vi "ME_acquire_16_DeltaForce_Daq.vi"() -> ()   [LabVIEW 2015]
doc: "Use this template to build a producer/consumer design pattern. Use this template when you need to execute a process, such as data analysis, when a data source, such as a triggered acquisition, produces data at an uneven rate and you need to execute the process when the data becomes available."
uses:
  Mode.ctl
  oxford_driver/Oxford Drivers/BUSGEN.LLB/OxfordAddress.ctl
  <vilib>/Analysis/baseanly.llb/Mean (DBL).vi
  <vilib>/DAQmx/read.llb/DAQmx Read (Analog 1D DBL 1Chan NSamp).vi
  <vilib>/DAQmx/create/channels.llb/DAQmx Create Channel (AI-Voltage-Basic).vi
  <vilib>/DAQmx/configure/timing.llb/DAQmx Timing (Sample Clock).vi
  <vilib>/Utility/file.llb/Write Delimited Spreadsheet (DBL).vi
  <vilib>/DAQmx/miscellaneous.llb/DAQmx Fill In Error Info.vi
  <vilib>/express/express arith-compare/Formula/XNode/ExpressFormulaBlockNode.xnode
  <vilib>/Analysis/NI_AALBase.lvlib
panel:
  out "T array":dbl[](array[numeric])
  out "Averaged I(T)":dbl[][](array[numeric])
  in  "Averaged P(T)":dbl[][](array[numeric])
  out "remaining elements 2":T1(array[cluster])
  out "Actual mean":dbl format="%0.6f"
  in  "Averaged dt":dbl[][](array[numeric])
  in  "Averaged P(B)":dbl[][](array[numeric])
  out "LockInR":dbl
  out "deltaUaux":dbl
  out "Actual Voltage (V)":dbl caption="Actual AuxV" step=0.1
  in  "Stop":bool
  out "SaveSweep":bool=TRUE
  out "Measurement File_dn":path
  out "Measurement File_up":path
  out "Measurement File_average":path
  out "Actual Polarization":dbl
  in  "Reset IB?":bool
  in  "First?":bool
  in  "Save Period":dbl=1.0
  out "Averaged I(B)":dbl[][](array[numeric])
  out "P(uC/mm^2)":dbl[](array[numeric])
  in  "Sweep":bool
  out "Offset array":dbl[](array[numeric])
  in  "stop 2":bool
  in  "dB":dbl=0.005
  out "appended array":dbl[][](array[numeric])
  out "Actual B Field (T)":dbl
  out "Actual Temperature (K)":dbl
  out "Actual Current (pA)":dbl
  in  "Tab Control":T2(tab)
  in  "dt (K)":dbl=0.1
  in  "Max temperature (K)":dbl=20.0
  in  "Min Temperature (K)":dbl=4.5
  out "P(T)":cluster{"yi":dbl[], dbl[]}(graph)
  out "I(T)":cluster{dbl[], dbl[]}(graph)
  in  "Set temperature (K)":dbl=4.5
  in  "Temp Ramping Rate (K/min)":dbl=10.0
  in  "Heater Range":enum16{"Off", "Low", "Medium", "High"}(ring)
  in  "Heater On/Off":bool
  out "Setpoint Temperature (K)":dbl
  out "I(T) /Averaged/":cluster{"B array":dbl[], dbl[]}[](graph)
  out "P(T) /Averaged/":cluster{"B array":dbl[], dbl[]}[](graph)
  out "Up/Down 2":bool
  out "I(B) 3":cluster{dbl[], dbl[]}[](graph)
  out "I(B) /Averaged/":cluster{"B array":dbl[], dbl[]}[](graph)
  out "P(B) /Averaged/":cluster{"B array":dbl[], dbl[]}[](graph)
  out "P(B)":cluster{"yi":dbl[], dbl[]}(graph)
  in  "Set Field (T)":dbl
  in  "Go to Set":bool
  in  "Sweep Rate (T/min)":dbl=2.0 format="%.6f"
  in  "Field To Zero":bool
  out "Target Field":dbl
  in  "Min Field (T)":dbl
  in  "Max Field (T)":dbl=0.15
  in  "Threshold B (T)":dbl
  out "Up/Down":bool
  in  "Magnetic Field array (T)":dbl[](array[numeric])=[0.025, 0.05, 0.075, 0.1, 0.125, 0.15, 0.175, 0.2, 0.225, 0.25, 0.275, 0.3]
  in  "T Sweep Rate Array":dbl[](array[numeric])=[10.0, 20.0]
  in  "Max count array":i32[](array[numeric])=[2, 1, 0, 0, 0, 9, 10, 11, 12]
  in  "secs to wait":dbl=180.0
  out "Wait (s)":dbl
  in  "Directory":string
  out "Finished":bool=TRUE
  out "Step Rate":bool
  out "New":bool=TRUE
  in  "Temperature Array":dbl[](array[numeric])=[4.5, 5.0, 6.0, 7.0, 8.0, 9.0, 10.0, 11.0, 12.0]
  in  "Sweep Rate Array":dbl[](array[numeric])=[2.0, 1.0, 0.5, 0.1, 0.05, 9.0, 10.0, 11.0, 12.0]
  in  "Record ALL":bool
  in  "Max Countl":i32
  out "i":i32
  out "j":i32
  out "Step Temp":bool
  in  "FileName":string
  in  "Measure Noise":bool
  in  "Cycles":i32
  in  "maximum value":dbl=10.0 format="%0.2f"
  in  "minimum value":dbl=-10.0 format="%0.2f"
  in  "physical channels":tag="Dev1/ai1"
  out "PSD (pA/Hz^1/2) Peaks Removed":cluster{"f0":dbl, "df":dbl, "magnitude":dbl[]}(graph)
  out "PSD (pA/Hz^1/2)":cluster{"f0":dbl, "df":dbl, "magnitude":dbl[]}(graph)
  out "Current (pA) Filtered":waveform(dbl)(graph)
  out "Current (pA)":dbl[](graph)
  in  "Samples per channel":i32=1000
  in  "Rate":dbl=1000.0 format="%0.2f"
  in  "Cut-Off Frequency":dbl=100.0 caption="Lower Cut-Off"
  in  "Filter On":bool
  in  "Keithley (IV conv) averaging":i32=10
  in  "Lock_in_Amplifier":refnum<visa-resource-name>="GPIB0::5::INSTR"
  out "Dc offset":dbl
  in  "Calibrate":bool
  in  "IV converter":refnum<visa-resource-name>="GPIB0::20::INSTR"
  in  "Magnetic Field":refnum<visa-resource-name>="GPIB0::21::INSTR"
  out "Time Lag":dbl=0.0500025749206543
  in  "Lake Shore":refnum<visa-resource-name>="GPIB0::11::INSTR"
  in  "Temp Refresh (s)":dbl=0.1
  in  "Sampling rate (Hz)":dbl=10.0
  in  "Gain (V/A)":dbl=1000000000.0
  in  "Sample area (mm^2)":dbl=1.0
  out "B_V":cluster{dbl[], "Best Linear Fit":dbl[]}[](graph)=[{[-0.00769241141, -0.00768011662, -0.0029394633, 0.00271952438, 0.00937200583, 0.0154641889, 0.0217080684, 0.0281692221, 0.0344763397, 0.0407091529, 0.0473661569, 0.0541476438, 0.0611164384, 0.0676637725, 0.073937413, 0.0801511723, 0.0863882257, 0.0933787866, 0.0997676928, 0.106163316, 0.113953626, 0.118979018, 0.126030157, 0.132855724, 0.13883398, 0.14631074, 0.153030676, 0.159156864, 0.165801088, 0.17248087, 0.178555009, 0.185285367, 0.192834407, 0.198751051, 0.205413053, 0.212847389, 0.219477697, 0.225574642, 0.232225854, 0.239015189, 0.245675966, 0.252411162, 0.258453848, 0.265211852, 0.271251534, 0.277801221, 0.284008329, 0.291402813, 0.297970768, 0.304082546, 0.310761405, 0.317366634, 0.323522001, 0.330123184, 0.336841279, 0.343557963, 0.349608435, 0.356238003, 0.363590921, 0.370338319, 0.376962983], "Best Linear Fit"=[0.0, 0.0015, 0.0035, 0.0056, 0.0076, 0.0096, 0.0116, 0.0136, 0.0156, 0.0177, 0.0197, 0.0219, 0.0239, 0.0259, 0.0279, 0.0299, 0.032, 0.034, 0.036, 0.038, 0.04, 0.042, 0.0441, 0.046, 0.048, 0.05, 0.052, 0.054, 0.056, 0.058, 0.06, 0.0621, 0.0643, 0.0663, 0.0684, 0.0704, 0.0725, 0.0745, 0.0765, 0.0787, 0.0807, 0.0827, 0.0847, 0.0868, 0.0888, 0.0908, 0.0928, 0.0948, 0.0968, 0.0988, 0.1008, 0.1028, 0.1048, 0.1069, 0.1091, 0.1111, 0.1131, 0.1152, 0.1173, 0.1193, 0.1213]}, {[-0.00769241141, -0.00768011662, -0.0029394633, 0.00271952438, 0.00937200583, 0.0154641889, 0.0217080684, 0.0281692221, 0.0344763397, 0.0407091529, 0.0473661569, 0.0541476438, 0.0611164384, 0.0676637725, 0.073937413, 0.0801511723, 0.0863882257, 0.0933787866, 0.0997676928, 0.106163316, 0.113953626, 0.118979018, 0.126030157, 0.132855724, 0.13883398, 0.14631074, 0.153030676, 0.159156864, 0.165801088, 0.17248087, 0.178555009, 0.185285367, 0.192834407, 0.198751051, 0.205413053, 0.212847389, 0.219477697, 0.225574642, 0.232225854, 0.239015189, 0.245675966, 0.252411162, 0.258453848, 0.265211852, 0.271251534, 0.277801221, 0.284008329, 0.291402813, 0.297970768, 0.304082546, 0.310761405, 0.317366634, 0.323522001, 0.330123184, 0.336841279, 0.343557963, 0.349608435, 0.356238003, 0.363590921, 0.370338319, 0.376962983], "Best Linear Fit"=[0.002353460844818253, 0.002357267374965663, 0.003824997997530172, 0.005577049655813272, 0.007636692089275871, 0.009522863265806463, 0.01145600043639222, 0.013456406815525209, 0.015409122826751182, 0.01733883381400479, 0.019399876452181594, 0.021499459635718428, 0.023657034245452215, 0.025684122519169482, 0.027626473848249778, 0.02955028565017564, 0.03148130942513291, 0.03364562299316916, 0.03562366117513693, 0.037603778974812686, 0.040015698972850115, 0.04157158615356273, 0.04375465501257369, 0.04586788562152819, 0.0477187843918964, 0.050033627699098075, 0.05211415440778254, 0.05401085368533849, 0.056067939569859164, 0.05813603439385595, 0.06001661903361471, 0.06210037244704129, 0.06443759401357516, 0.0662694173922171, 0.06833200743687069, 0.07063371605572277, 0.07268649347515121, 0.0745741389696738, 0.07663338837489471, 0.07873540137051047, 0.08079761214887074, 0.08288286343195213, 0.08475371006132383, 0.08684602281837933, 0.08871593939391825, 0.09074375613756333, 0.09266550866283872, 0.09495487889775463, 0.09698835150804998, 0.09888058937557581, 0.10094839843403076, 0.10299341126621803, 0.10489914451207855, 0.10694290468187984, 0.10902286140750632, 0.11110238128028392, 0.11297563849525552, 0.11502818680688229, 0.1173046879946565, 0.11939371707962458, 0.12144474708765744]}]
  out "V_I":cluster{dbl[], "Best Linear Fit":dbl[]}[](graph)=[{[0.0, 0.012, 0.026, 0.04, 0.054, 0.068, 0.081, 0.096, 0.11, 0.124, 0.138, 0.153, 0.167, 0.18, 0.195, 0.208, 0.223, 0.236, 0.251, 0.265, 0.279, 0.292, 0.306, 0.32, 0.334, 0.348, 0.362, 0.375, 0.389, 0.403, 0.417, 0.432, 0.446, 0.46, 0.475, 0.489, 0.504, 0.517, 0.531, 0.546, 0.56, 0.574, 0.588, 0.602, 0.616, 0.63, 0.644, 0.658, 0.672, 0.685, 0.699, 0.713, 0.727, 0.742, 0.755, 0.77, 0.784, 0.799, 0.814, 0.827, 0.841], "Best Linear Fit"=[-0.00769241141, -0.00768011662, -0.0029394633, 0.00271952438, 0.00937200583, 0.0154641889, 0.0217080684, 0.0281692221, 0.0344763397, 0.0407091529, 0.0473661569, 0.0541476438, 0.0611164384, 0.0676637725, 0.073937413, 0.0801511723, 0.0863882257, 0.0933787866, 0.0997676928, 0.106163316, 0.113953626, 0.118979018, 0.126030157, 0.132855724, 0.13883398, 0.14631074, 0.153030676, 0.159156864, 0.165801088, 0.17248087, 0.178555009, 0.185285367, 0.192834407, 0.198751051, 0.205413053, 0.212847389, 0.219477697, 0.225574642, 0.232225854, 0.239015189, 0.245675966, 0.252411162, 0.258453848, 0.265211852, 0.271251534, 0.277801221, 0.284008329, 0.291402813, 0.297970768, 0.304082546, 0.310761405, 0.317366634, 0.323522001, 0.330123184, 0.336841279, 0.343557963, 0.349608435, 0.356238003, 0.363590921, 0.370338319, 0.376962983]}, {[0.0, 0.012, 0.026, 0.04, 0.054, 0.068, 0.081, 0.096, 0.11, 0.124, 0.138, 0.153, 0.167, 0.18, 0.195, 0.208, 0.223, 0.236, 0.251, 0.265, 0.279, 0.292, 0.306, 0.32, 0.334, 0.348, 0.362, 0.375, 0.389, 0.403, 0.417, 0.432, 0.446, 0.46, 0.475, 0.489, 0.504, 0.517, 0.531, 0.546, 0.56, 0.574, 0.588, 0.602, 0.616, 0.63, 0.644, 0.658, 0.672, 0.685, 0.699, 0.713, 0.727, 0.742, 0.755, 0.77, 0.784, 0.799, 0.814, 0.827, 0.841], "Best Linear Fit"=[-0.015941127780698654, -0.010342478990544012, -0.0038107220686969304, 0.0027210348531501527, 0.009252791774997235, 0.01578454869684432, 0.02184975155284518, 0.028848062540538483, 0.03537981946238557, 0.041911576384232645, 0.048443333306079736, 0.05544164429377303, 0.061973401215620116, 0.06803860407162098, 0.07503691505931429, 0.08110211791531513, 0.08810042890300844, 0.0941656317590093, 0.10116394274670261, 0.1076956996685497, 0.11422745659039678, 0.12029265944639762, 0.1268244163682447, 0.1333561732900918, 0.13988793021193888, 0.14641968713378595, 0.15295144405563305, 0.15901664691163392, 0.165548403833481, 0.1720801607553281, 0.17861191767717516, 0.18561022866486845, 0.19214198558671555, 0.19867374250856262, 0.20567205349625592, 0.212203810418103, 0.2192021214057963, 0.22526732426179719, 0.23179908118364426, 0.23879739217133758, 0.24532914909318465, 0.2518609060150317, 0.2583926629368788, 0.2649244198587259, 0.271456176780573, 0.27798793370242003, 0.28451969062426713, 0.29105144754611423, 0.2975832044679613, 0.3036484073239622, 0.31018016424580924, 0.3167119211676563, 0.3232436780895034, 0.3302419890771967, 0.3363071919331976, 0.3433055029208909, 0.34983725984273795, 0.35683557083043127, 0.36383388181812454, 0.3698990846741254, 0.3764308415959725]}]
  out "B0 (T)":dbl=0.0026443907573365636
  out "B/V (T/V)":dbl=0.3027997253900218
  out "I0 (A)":dbl=-0.008736391445912099
  out "V/I (Ohm)":dbl=0.4773805959957447
  in  "Offset?":bool
  in  "Magnet":bool=TRUE
  in  "Ramp":bool=TRUE
  in  "DaQ":bool
  in  "Moving average":i8=10
  in  "Sample Rate":dbl=1000.0
  in  "Number of Samples":i32=100
  in  "Physical Channel":tag="kartya/ai0"
  in  "Min Voltage":dbl=-5.0
  in  "Max Voltage":dbl=5.0
  in  "Terminal Configuration":i32(ring)=-1 items=["default"=-1, "RSE"=10083, "NRSE"=10078, "Differential"=10106, "Pseudodifferential"=12529]
  out "Confirm":bool
  in  "Dwell Time (ms)":u32=1000
  in  "Temp/Magnetic Field":bool
  out "index":i8
  out "Read?":bool
  out "Magnetic Field (T)":dbl[](array[numeric])
  out "Reset":bool
  out "Measured Current (pA)":dbl[](array[numeric])
  out "Elapsed Time (s)":dbl[](array[numeric])
  out "Start time":timestamp
  in  "Enum":T3=enum."Process"
  out "B array":dbl[](array[numeric])
  in  "dB (T)":dbl=0.0025
  in  "Counter":i8
  out "L magnet (H)":dbl
  out "R magnet (mOhm)":dbl
  out "Actual Current (R0)":dbl
  out "Actual Field (T)":dbl
  out "Temperature array":dbl[](array[numeric])
  in  "New Measurement File":bool
  out "Measurement File":path
  out "refnum out":refnum<file>
  in  "Measuring":bool
  in  "Measure /Pause":bool
  in  "stop":bool
  # "DeltaForce"
  # "Discrete"
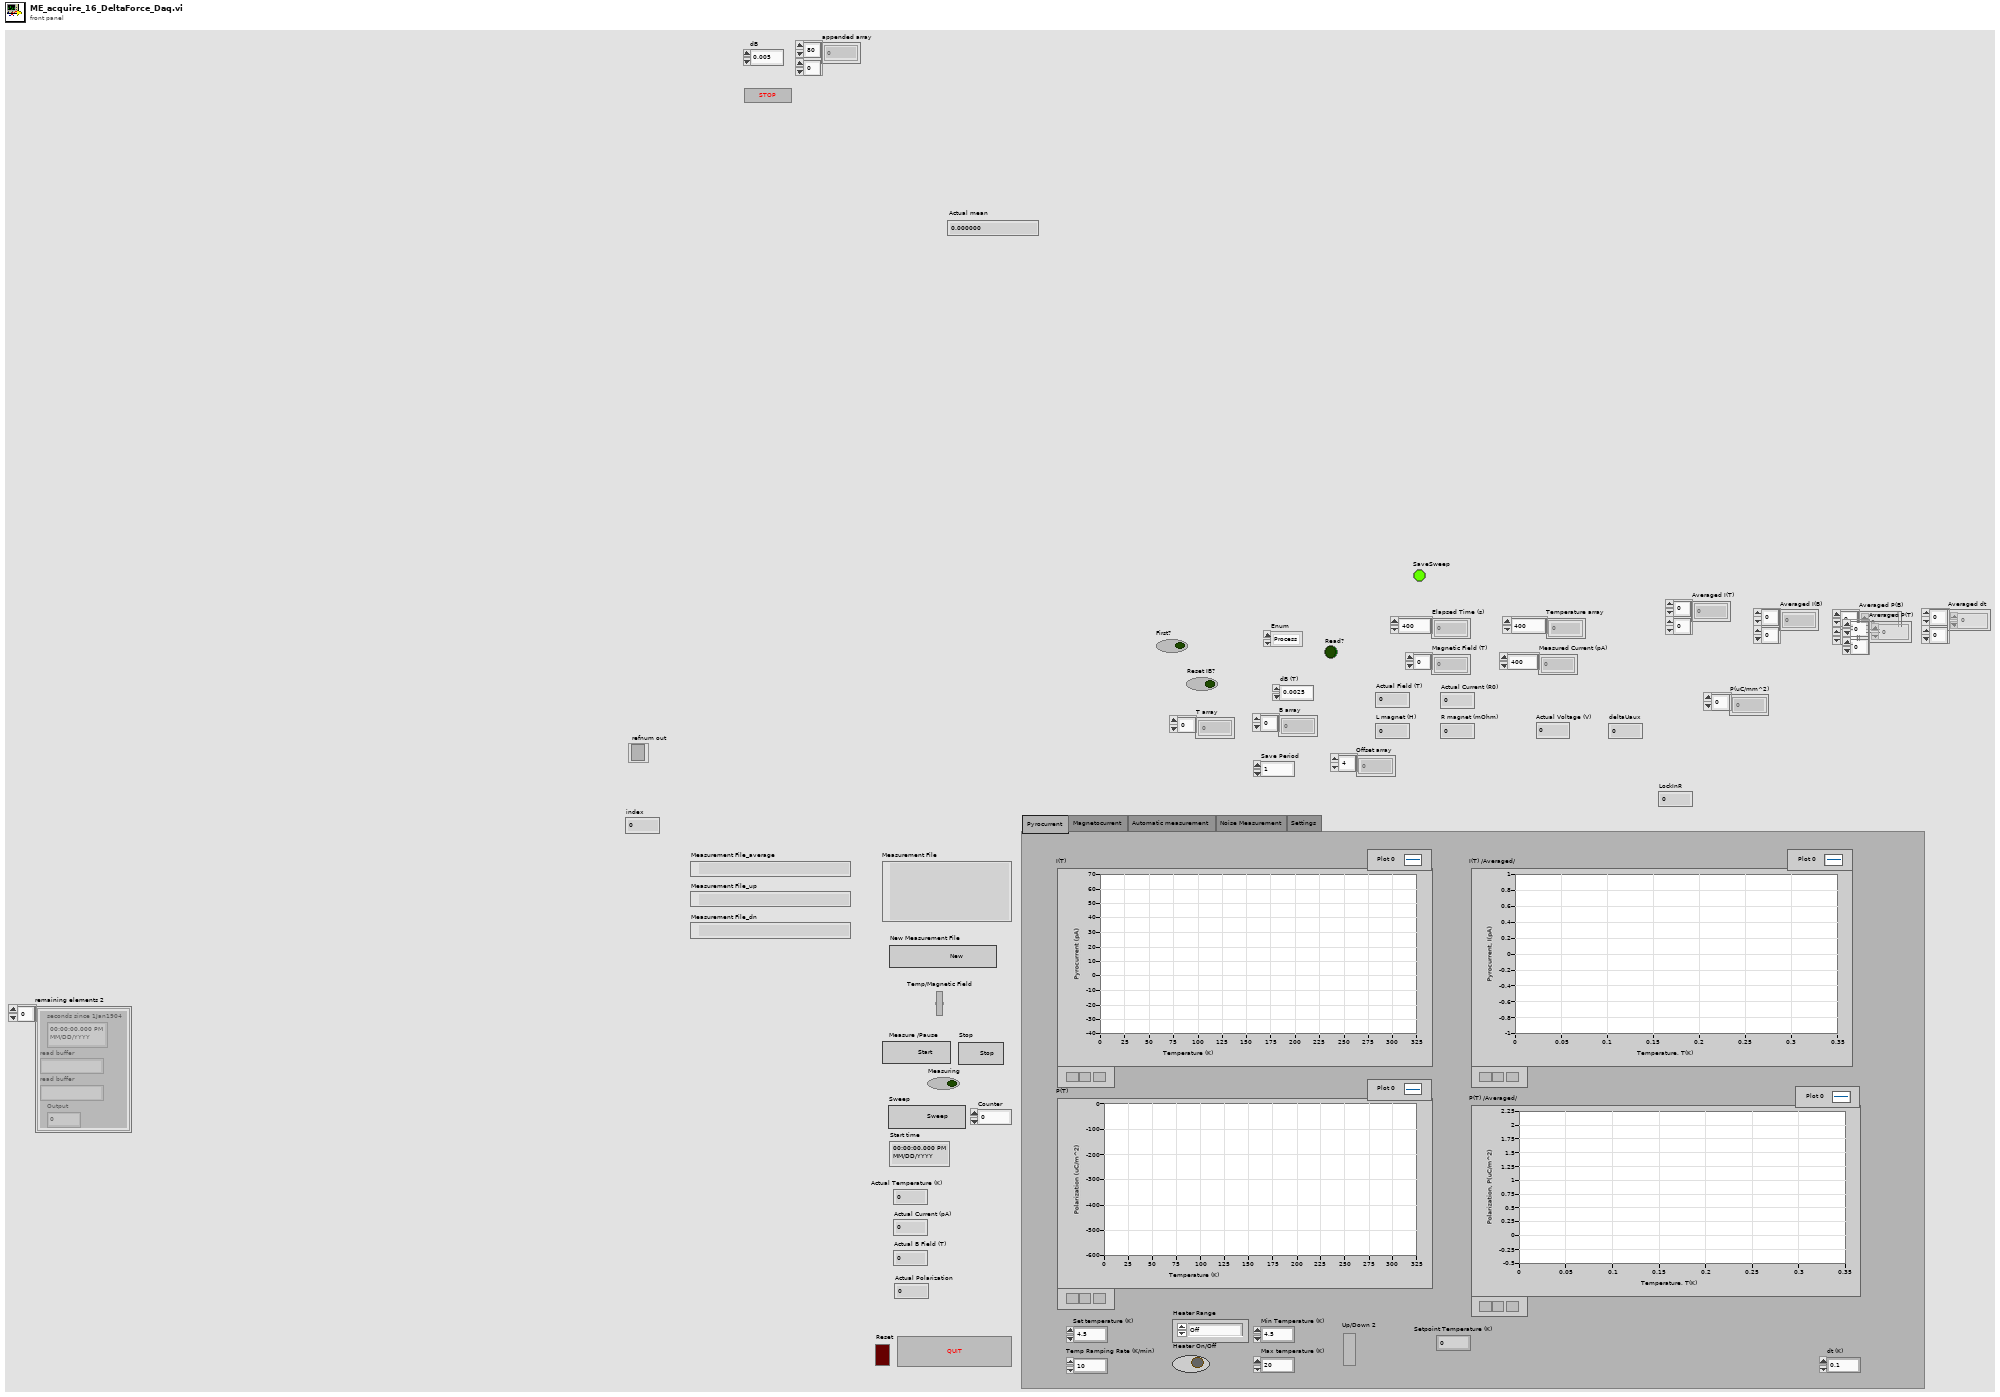
[diagram p1: front panel]
types:
  T1 = cluster{"seconds since 1Jan1904":timestamp, "read buffer":string, "read buffer":string, "Output":dbl}[]
  T2 = enum32{"Pyrocurrent", "Magnetocurrent", "Automatic measurement", "Noise Measurement", "Settings"}
  T3 = typedef "Mode.ctl" = enum16{"Offset", "Process", "Sweep", "StepOxford", "StepDelta", "Plot", "Save", "New", "Return", ""}
  T4 = cluster{"seconds since 1Jan1904":timestamp, "read buffer":string, "read buffer":string, "Output":dbl}
  T5 = enum16{"open", "replace", "create", "open or create", "replace or create", "replace or create with confirmation"}
  T6 = typedef "OxfordAddress.ctl" = cluster{"Com Port":i32, "ISOBUS Address":i32, "GPIB Address":i16, "Communication":enum16{"RS232", "ISOBUS", "GPIB", "Gateway"}}
  T7 = cluster{"B array":dbl[], "Averaged P(B) Out":dbl[]}
  T8 = cluster{"B array":dbl[], "BaselineSubtracted I(B)":dbl[]}
  T9 = cluster{"B array":dbl[], "Averaged P(B) Out":dbl[]}[]
  T10 = cluster{"B array":dbl[], "BaselineSubtracted I(B)":dbl[]}[]
  T11 = cluster{"T array":dbl[], "Averaged P(T) Out":dbl[]}
  T12 = cluster{"T array":dbl[], "Averaged I(B) out":dbl[]}
  T13 = cluster{"T array":dbl[], "Averaged P(T) Out":dbl[]}[]
  T14 = cluster{"T array":dbl[], "Averaged I(B) out":dbl[]}[]
  T15 = cluster{"I array out (A)":dbl[], "V array out (V)":dbl[]}
  T16 = cluster{"I array out (A)":dbl[], "Best Linear Fit":dbl[]}
  T17 = cluster{"V array out (V)":dbl[], "B array Out":dbl[]}
  T18 = cluster{"V array out (V)":dbl[], "Best Linear Fit 2":dbl[]}
  T19 = cluster{"I array out (A)":dbl[], "Best Linear Fit":dbl[]}[]
  T20 = cluster{"V array out (V)":dbl[], "Best Linear Fit 2":dbl[]}[]
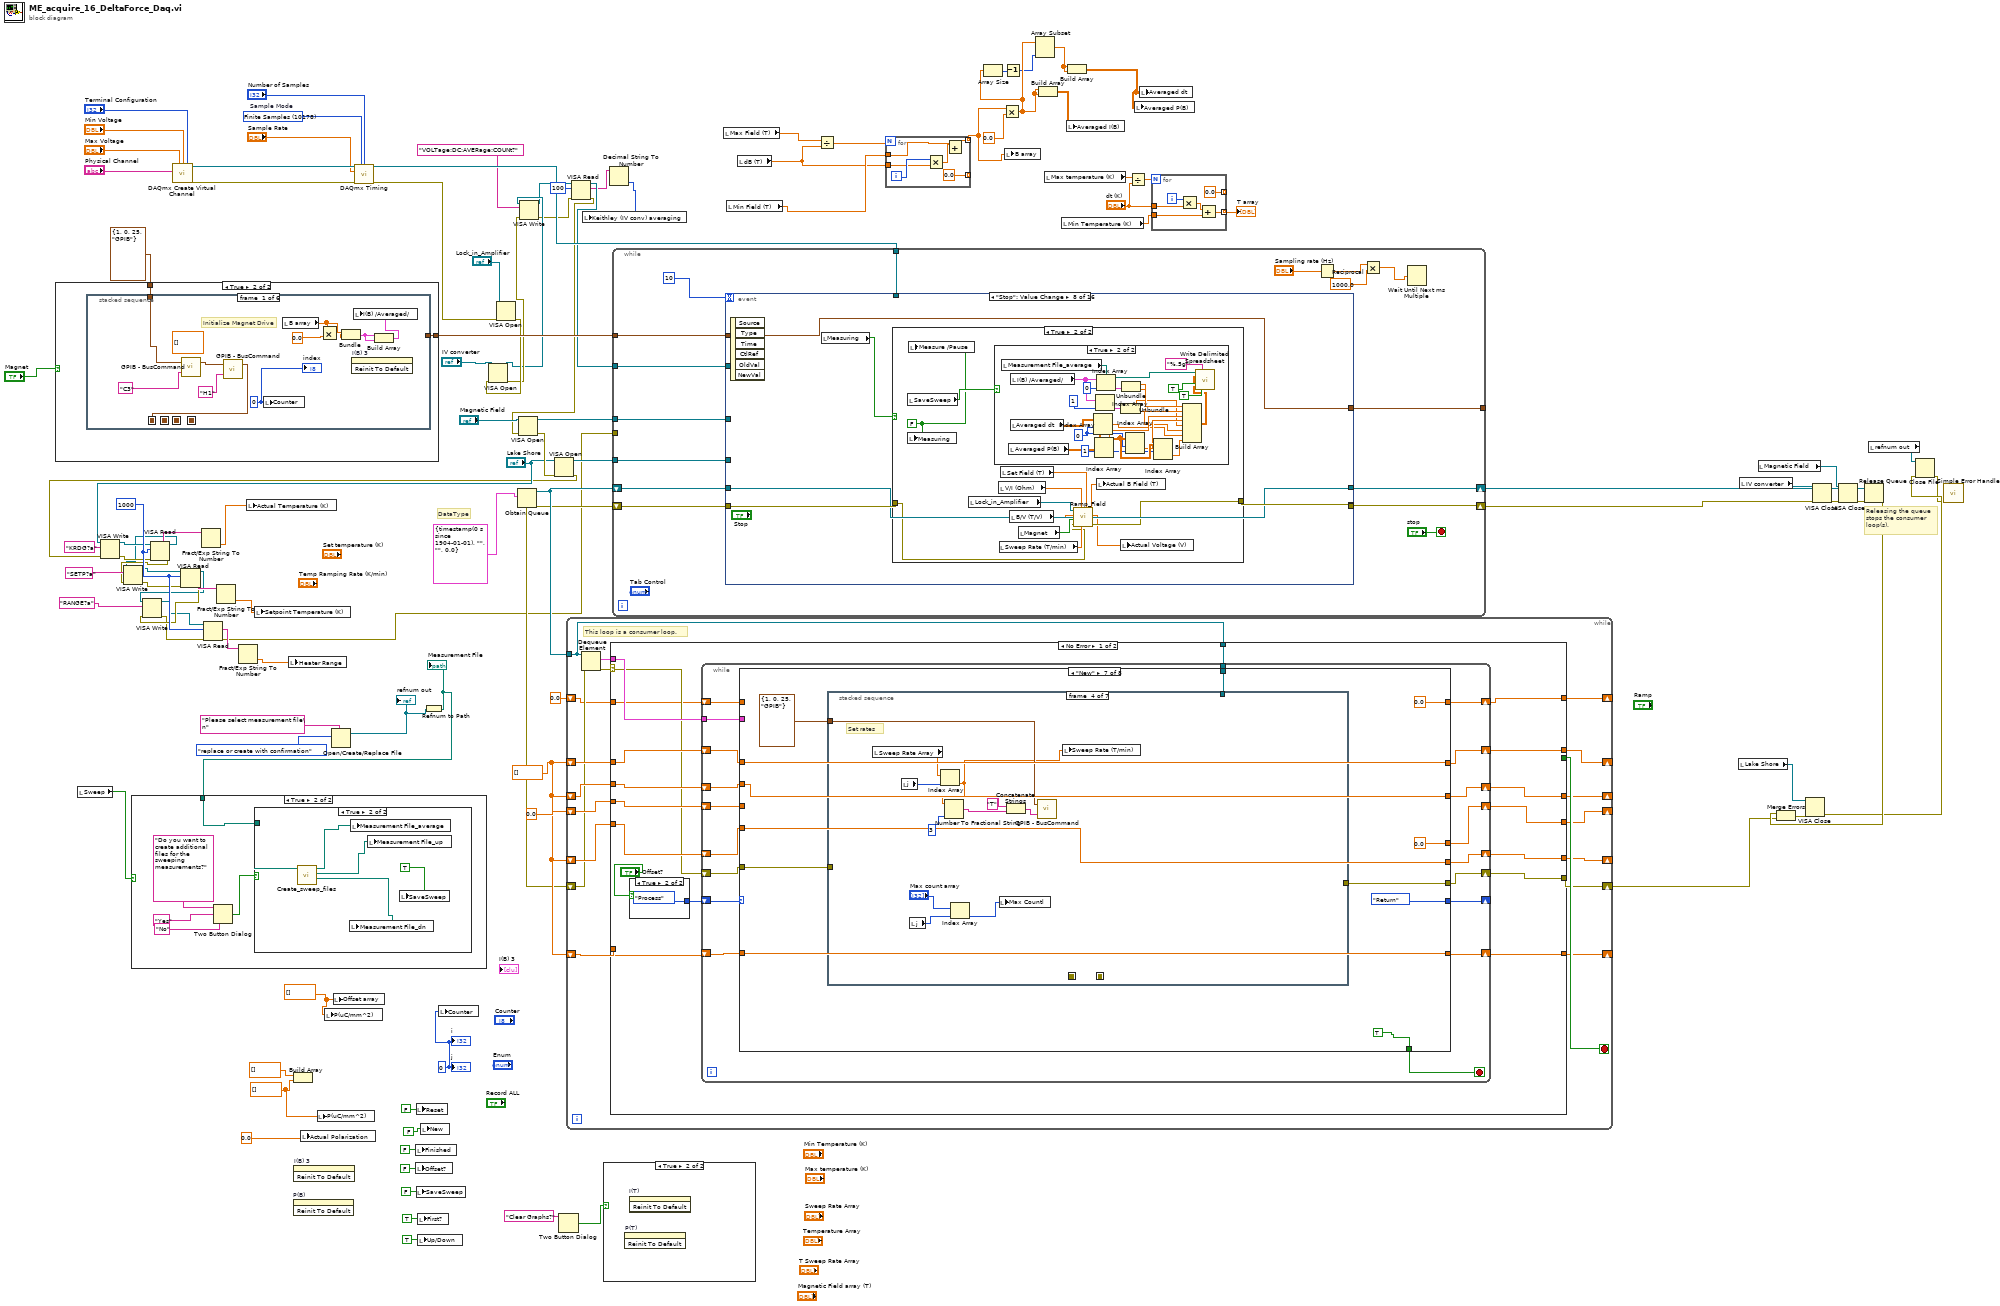
[diagram p0: block diagram]
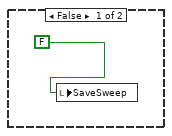
[diagram p4: hidden frame]
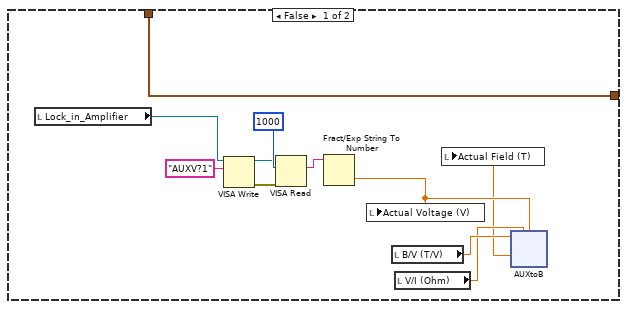
[diagram p5: hidden frame]
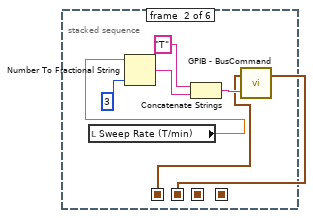
[diagram p6: hidden frame]
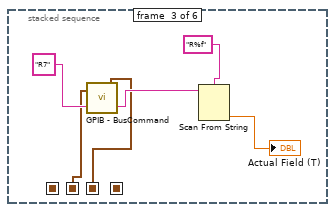
[diagram p7: hidden frame]
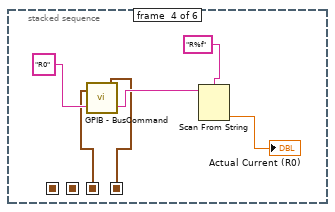
[diagram p8: hidden frame]
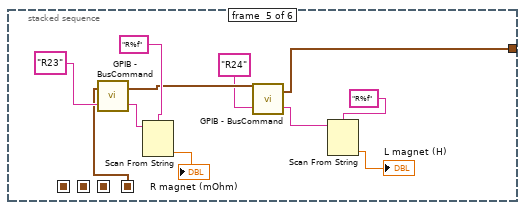
[diagram p9: hidden frame]
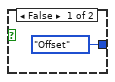
[diagram p11: hidden frame]
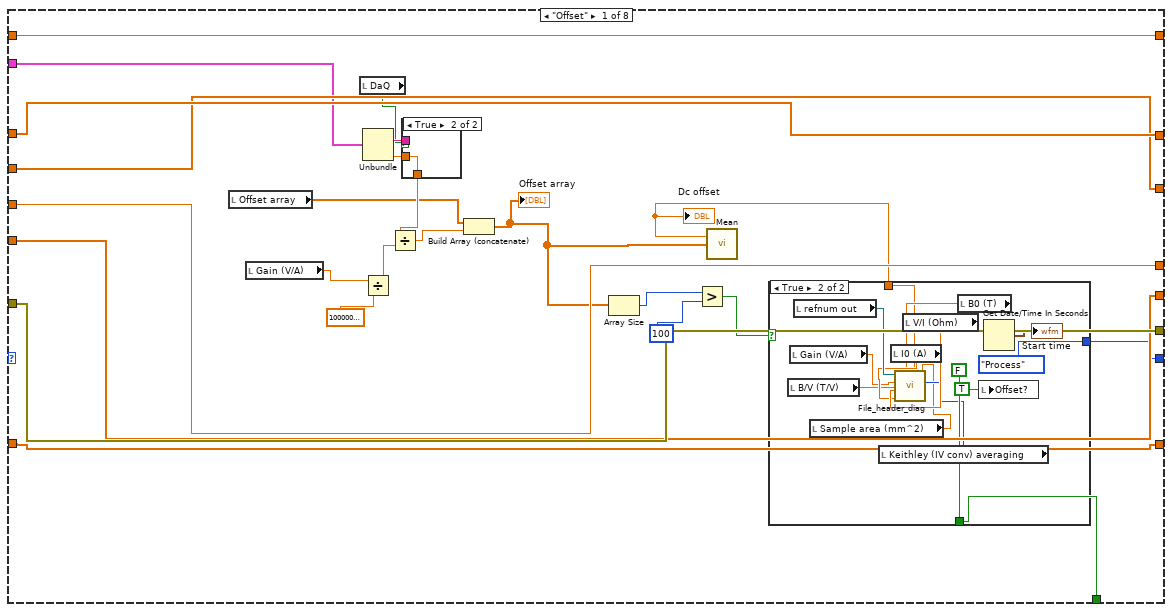
[diagram p12: hidden frame]
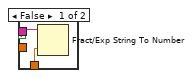
[diagram p13: hidden frame]
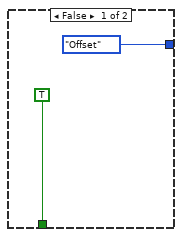
[diagram p14: hidden frame]
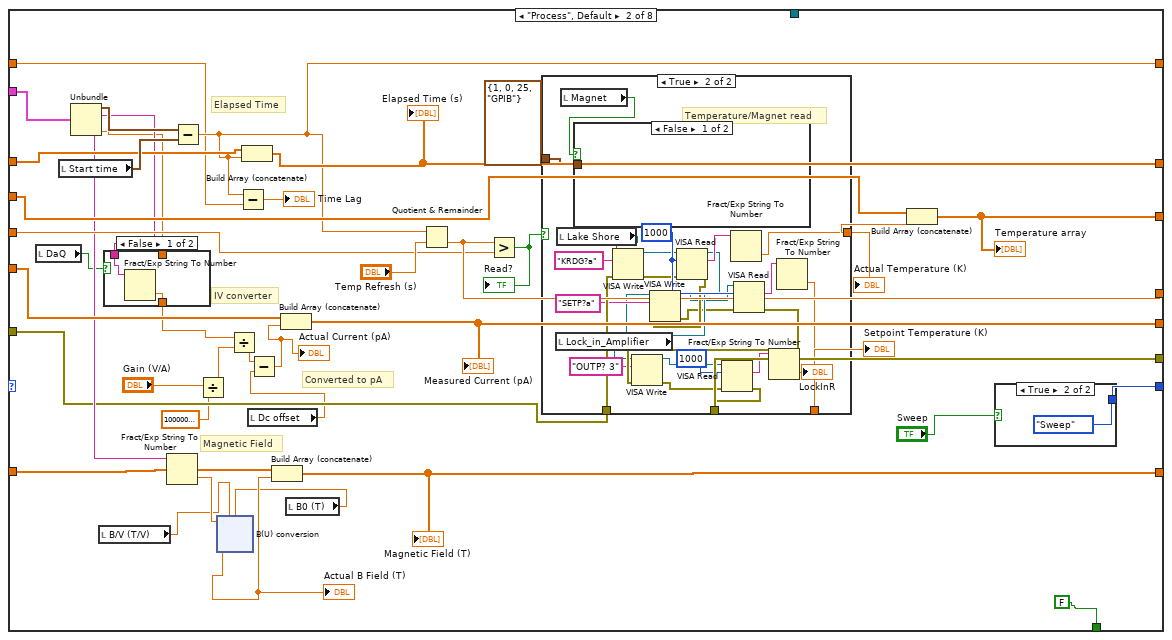
[diagram p15: hidden frame]
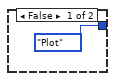
[diagram p17: hidden frame]
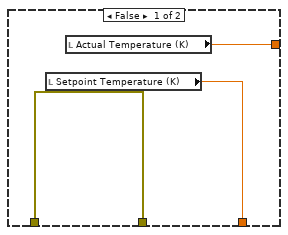
[diagram p18: hidden frame]
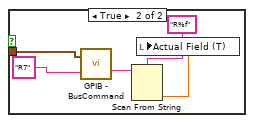
[diagram p19: hidden frame]
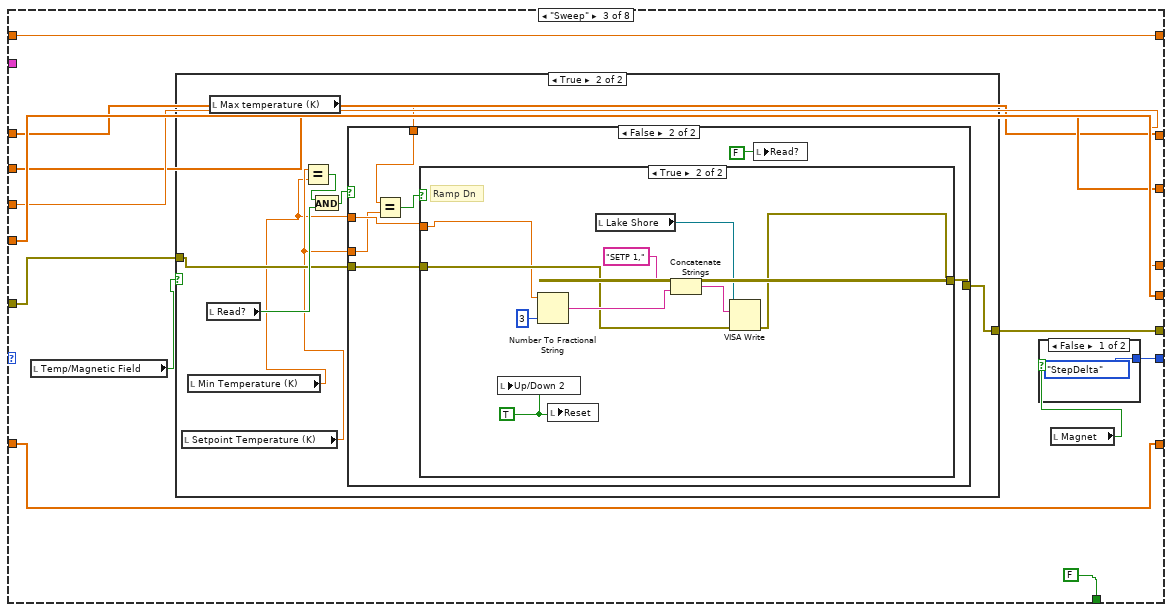
[diagram p20: hidden frame]
diagram:
  w27 = 10178 items=["Finite Samples"=10178, "Continuous Samples"=10123, "Hardware Timed Single Point"=12522]  # Sample Mode
  w54 = u32 1000 ("byte count")
  w65 = 0 ("j")
  w62 = dbl[] []
  w80 = dbl[] []
  w86 = dbl[] []
  # "DataType"
  # "Releasing the queue stops the consumer loop(s)."
  n1 = case shown="True" "Magnet" {
    tunnel: T6 {"Com Port"=1, "ISOBUS Address"=0, "GPIB Address"=25, "Communication"=enum."GPIB"} ("Address") -> [w120 w134]
    tunnel: [w120 w133] -> w92
    frame False {
      n2 = local read "Lock_in_Amplifier"() -> (w114:refnum<visa-resource-name>)
      n3 = VISA Write(VISA resource name=w114, write buffer="AUXV?1") -> (VISA resource name out=w115:refnum<visa-resource-name>, error out=w119:errorcluster)  [unwired: 1 in, 1 out]
      n4 = VISA Read(VISA resource name=w115, byte count=u32 1000, error in (no error)=w119) -> (read buffer=w118:string)  [unwired: 3 out]
      n5 = Fract/Exp String To Number(string=w118) -> (number=w111:dbl)  [unwired: 3 in, 1 out]
      n6 = local write "Actual Voltage (V)"(w111) -> ()
      n7 = local read "B/V (T/V)"() -> (w113:dbl)
      n8 = local read "V/I (Ohm)"() -> (w112:dbl)
      n9 = xnode "AUXtoB"("BpV"=w113, "Rm"=w112, "Aux"=w111) -> ("Result"=w110:dbl)  [unwired: 1 in, 1 out]
      n10 = local write "Actual Field (T)"(w110) -> ()
    }
    frame True {
      n11 = stacked-sequence {
        seq-local: [w142 _ _ _ _ _] -> [_ w147 _ _ _ _]
        seq-local: [_ w146 _ _ _ _] -> [_ _ w154 _ _ _]
        seq-local: [_ _ w153 _ _ _] -> [_ _ _ w160 _ _]
        seq-local: [_ _ _ w159 _ _] -> [_ _ _ _ w171 _]
        tunnel: w134 -> [w144 _ _ _ _ _]
        tunnel: [_ _ _ _ w169 _] -> w133
        frame #0 {
          (unwired) dbl[][] []
          w140 = i8 0 ("Counter")
          # "Initialize Magnet Drive"
          n12 = call "GPIB - BusCommand.vi"("Command"="C3", "Address"=w144) -> ("Address(thru)"=w143:T6)  [unwired: 1 out]
          n13 = call "GPIB - BusCommand.vi"("Command"="H1", "Address"=w143) -> ("Address(thru)"=w142:T6)  [unwired: 1 out]
          n14 = local write "Counter"(w140) -> ()
          n15 = local read "B array"() -> (w138:dbl[])
          n16 = Multiply(x=w138, y=0.0) -> (x*y=w137:dbl[])
          n17 = Bundle("B array"=w138, w137) -> (w136:cluster{"B array":dbl[], dbl[]})  [unwired: 1 in]
          n18 = invoke on="I(B) 3" class="XYGraph (strict)" method="Reinit To Default"() -> ()  [unwired: 3 in, 3 out]
          n19 = Build Array(w136, w136) -> (w135:cluster{"B array":dbl[], dbl[]}[])
          n20 = local write "I(B) /Averaged/"(w135) -> ()
          "index" <- w140
        }
        frame #1 {
          n21 = local read "Sweep Rate (T/min)"() -> (w148:dbl)
          n22 = Number To Fractional String(number=w148, precision (6)=i16 3) -> (F-format string=w150:string)  [unwired: 2 in]
          n23 = Concatenate Strings("T" ("format string"), w150) -> (w149:string)
          n24 = call "GPIB - BusCommand.vi"("Command"=w149, "Address"=w147) -> ("Address(thru)"=w146:T6)  [unwired: 1 out]
        }
        frame #2 {
          n25 = call "GPIB - BusCommand.vi"("Command"="R7" ("format string"), "Address"=w154) -> ("Reply"=w158:string, "Address(thru)"=w153:T6)
          n26 = Scan From String(format string="R%f" ("remaining string"), input string=w158) -> (output 1=→"Actual Field (T)":dbl)  [unwired: 3 in, 3 out]
        }
        frame #3 {
          n27 = call "GPIB - BusCommand.vi"("Command"="R0" ("format string"), "Address"=w160) -> ("Reply"=w164:string, "Address(thru)"=w159:T6)
          n28 = Scan From String(format string="R%f" ("remaining string"), input string=w164) -> (output 1=→"Actual Current (R0)":dbl)  [unwired: 3 in, 3 out]
        }
        frame #4 {
          n29 = call "GPIB - BusCommand.vi"("Command"="R23" ("format string"), "Address"=w171) -> ("Reply"=w175:string, "Address(thru)"=w170:T6)
          n30 = Scan From String(format string="R%f" ("remaining string"), input string=w175) -> (output 1=→"R magnet (mOhm)":dbl)  [unwired: 3 in, 3 out]
          n31 = call "GPIB - BusCommand.vi"("Command"="R24" ("format string"), "Address"=w170) -> ("Reply"=w167:string, "Address(thru)"=w169:T6)
          n32 = Scan From String(format string="R%f" ("remaining string"), input string=w167) -> (output 1=→"L magnet (H)":dbl)  [unwired: 3 in, 3 out]
        }
        frame #5 {
        }
      }
    }
  }
  n33 = local read "Sweep"() -> (w70:bool)
  n34 = call-poly <vilib>:"DAQmx Create Virtual Channel.vi"("maximum value"="Max Voltage", "minimum value"="Min Voltage", "input terminal configuration"="Terminal Configuration", "physical channels"="Physical Channel") -> ("task out"=w25:refnum<k21>, "error out"=w26:errorcluster)  [unwired: 10 in]
  n35 = Build Array(dbl[] [], w62) -> ()  [unwired: 1 out]
  n36 = invoke on="P(B)" class="XYGraph (strict)" method="Reinit To Default"() -> ()  [unwired: 3 in, 3 out]
  n37 = invoke on="I(B) 3" class="XYGraph (strict)" method="Reinit To Default"() -> ()  [unwired: 3 in, 3 out]
  n38 = local write "Actual Polarization"(0.0 ("Actual Polarization")) -> ()
  n39 = local write "P(uC/mm^2)"(w62) -> ()
  n40 = local write "P(uC/mm^2)"(w80) -> ()
  n41 = Open/Create/Replace File(prompt="Please select measurement file\n", operation (0:open)=T5."replace or create with confirmation") -> (refnum out=w89:refnum<file>)  [unwired: 4 in, 2 out]
  "refnum out" <- w89
  n42 = local write "Offset array"(w80) -> ()
  n43 = call-poly <vilib>:"DAQmx Timing.vi"("task/channels in"=w25, "sample mode"=w27, "samples per channel"="Number of Samples", "rate"="Sample Rate", "error in"=w26) -> ("task out"=w17:refnum<k21>, "error out"=w18:errorcluster)  [unwired: 9 in]
  n44 = local write "Finished"(FALSE ("Finished")) -> ()
  n45 = local write "Offset?"(FALSE ("Offset?")) -> ()
  n46 = local write "Reset"(FALSE ("Reset")) -> ()
  n47 = local write "SaveSweep"(FALSE ("SaveSweep")) -> ()
  n48 = local write "First?"(TRUE ("First?")) -> ()
  n49 = local write "Up/Down"(TRUE ("Up/Down")) -> ()
  n50 = local write "New"(FALSE ("New")) -> ()
  n51 = Refnum to Path(1:w89) -> (0:w69:path)
  "Measurement File" <- w69
  n52 = case shown="True" w70 {
    tunnel: w69 -> [_ w176]
    frame False {
    }
    frame True {
      n53 = Two Button Dialog(message="Do you want to create additional files for the sweeping measurements?" ("string"), 1:"No" ("F button name (\"Cancel\")"), 2:"Yes" ("T button name (\"OK\")")) -> (T button?=w178:bool)
      n54 = case shown="True" w178 {
        tunnel: w176 -> [_ w186]
        frame False {
          n55 = local write "SaveSweep"(FALSE ("SaveSweep")) -> ()
        }
        frame True {
          n56 = call "Create_sweep_files.vi"("Measurement File"=w186) -> ("Path 3"=w183:path, "Path 2"=w184:path, "Path"=w185:path)  [unwired: 8 in]
          n57 = local write "Measurement File_dn"(w183) -> ()
          n58 = local write "Measurement File_average"(w185) -> ()
          n59 = local write "Measurement File_up"(w184) -> ()
          n60 = local write "SaveSweep"(TRUE) -> ()
        }
      }
    }
  }
  n61 = local write "Counter"(w65) -> ()
  n62 = VISA Open(error in (no error)=w18, VISA resource name="Lock_in_Amplifier") -> (error out=w37:errorcluster)  [unwired: 3 in, 1 out]
  n63 = VISA Open(error in (no error)=w37, VISA resource name="IV converter") -> (VISA resource name=w14:refnum<visa-resource-name>, error out=w15:errorcluster)  [unwired: 3 in]
  n64 = Obtain Queue(element data type=T4 {"seconds since 1Jan1904"=timestamp(0 s since 1904-01-01), "read buffer"="", "read buffer"="", "Output"=0.0} ("output cluster")) -> (queue out=w109:refnum<queue>, error out=w84:errorcluster)  [unwired: 4 in, 1 out]
  n65 = VISA Write(VISA resource name=w14, write buffer="VOLTage:DC:AVERage:COUNt?", error in (no error)=w15) -> (VISA resource name out=w10:refnum<visa-resource-name>, error out=w12:errorcluster)  [unwired: 1 out]
  n66 = Two Button Dialog(message="Clear Graphs?") -> (T button?=w64:bool)  [unwired: 2 in]
  n67 = while {
    tunnel: w109 -> [w187]
    shift-right: [w200] -> _
    shift-left: w86 -> [w199]
    shift-right: [w198] -> _
    shift-left: w86 -> [w197]
    shift-right: [w196] -> _
    shift-left: w86 -> [w195]
    shift-right: [w194] -> _
    shift-left: 0.0 -> [w193]
    shift-right: [w192] -> _
    shift-left: w86 -> [w191]
    shift-right: [w201] -> w97
    shift-left: w84 -> [w190]
    shift-right: [w189] -> _
    shift-left: 0.0 -> [w188]
    stop <- w202 stop-if-true
    # "This loop is a consumer loop."
    n68 = Dequeue Element(queue=w187, error in (no error)=w190) -> (element=w203:T4, error out=w204:errorcluster)  [unwired: 1 in, 2 out]
    n69 = case shown="No Error" w204 {
      selector: w204 -> [w210 w934]
      tunnel: w203 -> [w221 _]
      tunnel: [_ TRUE] -> w202
      tunnel: [w209 w934] -> w201
      tunnel: [w220 w933] -> w200
      tunnel: w199 -> [w219 w933]
      tunnel: [w218 w930] -> w198
      tunnel: w197 -> [w217 w930]
      tunnel: [w216 w929] -> w196
      tunnel: w195 -> [w215 w929]
      tunnel: [w214 w931] -> w194
      tunnel: w193 -> [w213 w931]
      tunnel: [w212 w932] -> w192
      tunnel: w191 -> [w211 w932]
      tunnel: [w208 w928] -> w189
      tunnel: w188 -> [w207 w928]
      tunnel: w187 -> [w205 _]
      frame No Error {
        n70 = case shown="True" "Offset?" {
          tunnel: [Mode."Offset" ("Enum") Mode."Process" ("Enum")] -> w222
          frame False {
          }
          frame True {
          }
        }
        n71 = while {
          shift-right: [w231] -> _
          shift-left: w222 -> [w243]
          tunnel: w221 -> [w242]
          shift-right: [w241] -> w220
          shift-left: w219 -> [w240]
          shift-right: [w233] -> w212
          shift-left: w211 -> [w232]
          shift-right: [w235] -> w214
          shift-left: w213 -> [w234]
          shift-right: [w239] -> w218
          shift-left: w217 -> [w238]
          shift-right: [w229] -> w209
          shift-left: w210 -> [w230]
          shift-right: [w237] -> w216
          shift-left: w215 -> [w236]
          shift-right: [w227] -> w208
          shift-left: w207 -> [w226]
          tunnel: w205 -> [w225]
          stop <- w228 stop-if-true
          n72 = case shown="\"New\"" w243 {
            selector: w243 -> [_ _ _ _ _ _ _ w921]
            tunnel: w242 -> [w261 w324 _ _ _ _ _ _]
            tunnel: [w267 w321 w382 w516 w578 w651 w762 w926] -> w241
            tunnel: w240 -> [w267 w314 w382 w516 w578 w647 w762 w926]
            tunnel: [w262 w320 w385 w513 w580 w653 w760 w923] -> w239
            tunnel: w238 -> [w262 w319 w385 w513 w580 w648 w760 w923]
            tunnel: [w263 w318 w387 w511 w575 w654 w758 w920] -> w237
            tunnel: w236 -> [w263 w317 w387 w511 w575 w649 w758 w920]
            tunnel: [w265 w313 w384 w514 w576 w657 0.0 w924] -> w235
            tunnel: w234 -> [w265 w312 w384 w514 w576 w657 _ w924]
            tunnel: [w266 w309 w383 w515 w577 w652 w761 w925] -> w233
            tunnel: w232 -> [w266 w310 w383 w515 w577 w650 w761 w925]
            tunnel: [w250 w307 w380 Mode."Plot" ("Enum") Mode."Save" ("Enum") w658 Mode."Return" ("Enum") w921] -> w231
            tunnel: w230 -> [w264 w305 w389 w508 w583 w656 w754 w922]
            tunnel: [w264 w304 w388 w507 w583 w656 w753 w922] -> w229
            tunnel: [w246 FALSE FALSE FALSE FALSE w645 TRUE TRUE] -> w228
            tunnel: [w249 w301 w381 w509 w579 w655 0.0 w927] -> w227
            tunnel: w226 -> [w249 w300 w381 w509 w579 w655 _ w927]
            tunnel: w225 -> [_ _ _ _ _ _ w752 _]
            frame "Offset" {
              n73 = local read "Offset array"() -> (w255:dbl[])
              n74 = local read "Gain (V/A)"() -> (w259:dbl)
              n75 = local read "DaQ"() -> (w245:bool)
              n76 = Unbundle(w261) -> ("read buffer"=w248:string, "Output"=w244:dbl)  [unwired: 2 out]
              n77 = Divide(x=w259, y=1000000000000.0) -> (x/y=w257:dbl)
              n78 = case shown="True" w245 {
                tunnel: [w269 w270] -> w260
                tunnel: w248 -> [w268 _]
                tunnel: w244 -> [_ w270]
                frame False {
                  n79 = Fract/Exp String To Number(string=w268) -> (number=w269:dbl)  [unwired: 3 in, 1 out]
                }
                frame True {
                }
              }
              n80 = Divide(x=w260, y=w257) -> (x/y=w256:dbl)
              n81 = Build Array (concatenate)(w255, w256) -> (w251:dbl[])
              "Offset array" <- w251
              n82 = Array Size(array=w251) -> (size(s)=w254:i32)
              n83 = Greater?(x=w254, y=100) -> (0:w252:bool)
              n84 = call-poly <vilib>:"Mean.vi"("X"=w251) -> ("mean"=w247:dbl)  [unwired: 1 out]
              "Dc offset" <- w247
              n85 = case shown="True" w252 {
                tunnel: [Mode."Offset" ("Enum") Mode."Process" ("Enum")] -> w250
                tunnel: w247 -> [_ w277]
                tunnel: [TRUE FALSE] -> w246
                frame False {
                }
                frame True {
                  n86 = local read "B/V (T/V)"() -> (w278:dbl)
                  n87 = local read "Gain (V/A)"() -> (w279:dbl)
                  n88 = local read "refnum out"() -> (w283:refnum<file>)
                  n89 = local read "Sample area (mm^2)"() -> (w273:dbl)
                  n90 = local read "Keithley (IV conv) averaging"() -> (w274:i32)
                  n91 = local read "I0 (A)"() -> (w281:dbl)
                  n92 = local read "V/I (Ohm)"() -> (w282:dbl)
                  n93 = local read "B0 (T)"() -> (w280:dbl)
                  n94 = call "File_header_diag.vi"("Averaging"=w274, "Sample area"=w273, "OFFSET"=w277, "B0"=w280, "B/V"=w278, "I0"=w281, "V/I"=w282, "Gain"=w279, "Byte Stream File in"=w283) -> ()  [unwired: 3 in]
                  n95 = local write "Offset?"(TRUE ("Offset?")) -> ()
                  n96 = Get Date/Time In Seconds() -> (seconds since 1Jan1904=→"Start time":timestamp)
                }
              }
            }
            frame "Process", Default {
              # "Converted to pA"
              # "Magnetic Field"
              # "IV converter"
              # "Elapsed Time"
              n97 = local read "DaQ"() -> (w288:bool)
              n98 = local read "Start time"() -> (w322:timestamp)
              n99 = Unbundle(w324) -> ("seconds since 1Jan1904"=w323:timestamp, "read buffer"=w289:string, "read buffer"=w306:string, "Output"=w286:dbl)
              n100 = local read "B/V (T/V)"() -> (w296:dbl)
              n101 = case shown="False" w288 {
                tunnel: w289 -> [w328 _]
                tunnel: [w327 w329] -> w287
                tunnel: w286 -> [_ w329]
                frame False {
                  n102 = Fract/Exp String To Number(string=w328) -> (number=w327:dbl)  [unwired: 3 in, 1 out]
                }
                frame True {
                }
              }
              n103 = Fract/Exp String To Number(string=w306) -> (number=w316:dbl)  [unwired: 3 in, 1 out]
              n104 = Subtract(x=w323, y=w322) -> (x-y=w301:dbl)
              n105 = Divide(x="Gain (V/A)", y=1000000000000.0) -> (x/y=w299:dbl)
              n106 = Divide(x=w287, y=w299) -> (x/y=w294:dbl)
              n107 = Subtract(x=w301, y=w300) -> (x-y=→"Time Lag":dbl)
              n108 = Build Array (concatenate)(w314, w301) -> (w321:dbl[])
              "Elapsed Time (s)" <- w321
              n109 = local read "Dc offset"() -> (w292:dbl)
              n110 = Subtract(x=w294, y=w292) -> (x-y=w293:dbl)
              "Actual Current (pA)" <- w293
              n111 = Build Array (concatenate)(w319, w293) -> (w320:dbl[])
              "Measured Current (pA)" <- w320
              n112 = local read "B0 (T)"() -> (w295:dbl)
              n113 = xnode "B(U) conversion"("V"=w316, "BpV"=w296, "B0"=w295) -> ("Result"=w315:dbl)  [unwired: 1 in, 1 out]
              "Actual B Field (T)" <- w315
              n114 = Build Array (concatenate)(w317, w315) -> (w318:dbl[])
              "Magnetic Field (T)" <- w318
              n115 = Quotient & Remainder(x=w301, y="Temp Refresh (s)") -> (floor(x/y)=w313:dbl)  [unwired: 1 out]
              n116 = Greater?(x=w313, y=w312) -> (0:w311:bool)
              "Read?" <- w311
              n117 = case shown="True" w311 {
                tunnel: [w333 w358] -> w308
                tunnel: w305 -> [w334 w357]
                tunnel: [w334 w337] -> w304
                tunnel: T6 {"Com Port"=1, "ISOBUS Address"=0, "GPIB Address"=25, "Communication"=enum."GPIB"} ("Address") -> [_ w356]
                tunnel: [w332 w352] -> w290
                frame False {
                  n118 = local read "Setpoint Temperature (K)"() -> (w332:dbl)
                  n119 = local read "Actual Temperature (K)"() -> (w333:dbl)
                }
                frame True {
                  w353 = u32 1000 ("byte count")
                  # "Temperature/Magnet read"
                  n120 = local read "Lock_in_Amplifier"() -> (w341:refnum<visa-resource-name>)
                  n121 = local read "Lake Shore"() -> (w355:refnum<visa-resource-name>)
                  n122 = local read "Magnet"() -> (w344:bool)
                  n123 = case shown="False" w344 {
                    tunnel: w356 -> [_ w362]
                    frame False {
                    }
                    frame True {
                      n124 = call "GPIB - BusCommand.vi"("Command"="R7" ("format string"), "Address"=w362) -> ("Reply"=w363:string)  [unwired: 1 out]
                      n125 = Scan From String(format string="R%f" ("remaining string"), input string=w363) -> (output 1=w361:dbl)  [unwired: 3 in, 3 out]
                      n126 = local write "Actual Field (T)"(w361) -> ()
                    }
                  }
                  n127 = VISA Write(VISA resource name=w355, write buffer="KRDG?a", error in (no error)=w357) -> (VISA resource name out=w351:refnum<visa-resource-name>, error out=w349:errorcluster)  [unwired: 1 out]
                  n128 = VISA Read(VISA resource name=w351, byte count=w353, error in (no error)=w349) -> (VISA resource name out=w350:refnum<visa-resource-name>, read buffer=w359:string, error out=w348:errorcluster)  [unwired: 1 out]
                  n129 = VISA Write(VISA resource name=w350, write buffer="SETP?a", error in (no error)=w348) -> (VISA resource name out=w346:refnum<visa-resource-name>, error out=w347:errorcluster)  [unwired: 1 out]
                  n130 = Fract/Exp String To Number(string=w359) -> (number=w358:dbl)  [unwired: 3 in, 1 out]
                  n131 = VISA Read(VISA resource name=w346, byte count=w353, error in (no error)=w347) -> (read buffer=w345:string, error out=w343:errorcluster)  [unwired: 2 out]
                  n132 = VISA Write(VISA resource name=w341, write buffer="OUTP? 3", error in (no error)=w343) -> (VISA resource name out=w340:refnum<visa-resource-name>, error out=w342:errorcluster)  [unwired: 1 out]
                  n133 = VISA Read(VISA resource name=w340, byte count=u32 1000, error in (no error)=w342) -> (read buffer=w336:string, error out=w337:errorcluster)  [unwired: 2 out]
                  n134 = Fract/Exp String To Number(string=w336) -> (number=→"LockInR":dbl)  [unwired: 3 in, 1 out]
                  n135 = Fract/Exp String To Number(string=w345) -> (number=w352:dbl)  [unwired: 3 in, 1 out]
                }
              }
              "Actual Temperature (K)" <- w308
              "Setpoint Temperature (K)" <- w290
              n136 = Build Array (concatenate)(w310, w308) -> (w309:dbl[])
              "Temperature array" <- w309
              n137 = case shown="True" "Sweep" {
                tunnel: [Mode."Plot" ("Enum") Mode."Sweep" ("Enum")] -> w307
                frame False {
                }
                frame True {
                }
              }
            }
            frame "Sweep" {
              n138 = local read "Temp/Magnetic Field"() -> (w379:bool)
              n139 = case shown="True" w379 {
                tunnel: w389 -> [w398 w455]
                tunnel: [w397 w454] -> w388
                frame False {
                  n140 = local read "Actual Field (T)"() -> (w393:dbl)
                  n141 = local read "Min Field (T)"() -> (w392:dbl)
                  n142 = local read "Max Field (T)"() -> (w399:dbl)
                  n143 = local read "Read?"() -> (w396:bool)
                  n144 = Greater Or Equal?(x=w392, y=w393) -> (x >= y?=w395:bool)
                  n145 = Compound Arithmetic op=AND(w395, w396) -> (w394:bool)
                  n146 = case shown="False" w394 {
                    tunnel: [w402 w438] -> w397
                    tunnel: w399 -> [w400 w437]
                    tunnel: w392 -> [_ w436]
                    tunnel: w393 -> [_ w434]
                    tunnel: w398 -> [w403 w433]
                    frame True {
                      # "Ramp Up"
                      n147 = case shown="True" "First?" {
                        tunnel: [TRUE ("Save") FALSE ("Save")] -> w406
                        tunnel: [w425 w429] -> w405
                        frame False {
                          n148 = local read "Counter"() -> (w428:i8)
                          n149 = local write "Actual Polarization"(0.0 ("Actual Polarization")) -> ()
                          n150 = Increment(x=w428) -> (x+1=w425:i8)
                          n151 = local write "Counter"(w425) -> ()
                        }
                        frame True {
                          n152 = local read "Counter"() -> (w429:i8)
                          n153 = local write "First?"(FALSE ("First?")) -> ()
                        }
                      }
                      "Reset" <- w406
                      n154 = local write "Read?"(FALSE ("Read?")) -> ()
                      n155 = local read "Record ALL"() -> (w401:bool)
                      n156 = case shown="True" w401 {
                        tunnel: w405 -> [_ w413]
                        tunnel: [FALSE w411] -> w404
                        frame False {
                        }
                        frame True {
                          n157 = Greater?(x=w413, y="Max Countl") -> (0:w411:bool)
                        }
                      }
                      n158 = case shown="True" w404 {
                        tunnel: w403 -> [w417 w424]
                        tunnel: [w416 w424] -> w402
                        tunnel: w400 -> [w415 _]
                        frame False {
                          n159 = local read "Magnet"() -> (w414:bool)
                          n160 = case shown="True" w414 {
                            tunnel: w417 -> [w418 w421]
                            tunnel: [w418 w420] -> w416
                            tunnel: w415 -> [_ w419]
                            frame False {
                            }
                            frame True {
                              n161 = call "Set_B.vi"("error in (no error)"=w421, "address string"="25", "Set Field (T)"=w419) -> ("error out"=w420:errorcluster)  [unwired: 8 in]
                            }
                          }
                          "Target Field" <- w415
                        }
                        frame True {
                          "New" <- TRUE
                        }
                      }
                      "Up/Down" <- FALSE ("Up/Down")
                    }
                    frame False {
                      n162 = Less Or Equal?(x=w437, y=w434) -> (x <= y?=w435:bool)
                      n163 = case shown="True" w435 {
                        tunnel: [w439 w443] -> w438
                        tunnel: w436 -> [_ w441]
                        tunnel: w433 -> [w439 w444]
                        frame False {
                        }
                        frame True {
                          # "Resetting at the end of every cycle"
                          # "Ramp Dn"
                          n164 = local write "Up/Down"(TRUE ("Up/Down")) -> ()
                          n165 = local read "Magnet"() -> (w440:bool)
                          n166 = local write "Target Field"(w441) -> ()
                          n167 = local write "Reset"(TRUE ("Reset")) -> ()
                          n168 = case shown="True" w440 {
                            tunnel: w444 -> [w446 w449]
                            tunnel: [w446 w448] -> w443
                            tunnel: w441 -> [_ w447]
                            frame False {
                            }
                            frame True {
                              n169 = call "Set_B.vi"("error in (no error)"=w449, "address string"="25", "Set Field (T)"=w447) -> ("error out"=w448:errorcluster)  [unwired: 8 in]
                            }
                          }
                        }
                      }
                      n170 = local write "Read?"(FALSE ("Read?")) -> ()
                    }
                  }
                }
                frame True {
                  n171 = local read "Setpoint Temperature (K)"() -> (w453:dbl)
                  n172 = local read "Min Temperature (K)"() -> (w452:dbl)
                  n173 = local read "Read?"() -> (w458:bool)
                  n174 = local read "Max temperature (K)"() -> (w451:dbl)
                  n175 = Equal?(x=w453, y=w452) -> (x = y?=w456:bool)
                  n176 = And(x=w456, y=w458) -> (x .and. y?=w457:bool)
                  n177 = case shown="False" w457 {
                    tunnel: [w459 w496] -> w454
                    tunnel: w451 -> [w467 w495]
                    tunnel: w452 -> [_ w494]
                    tunnel: w453 -> [_ w492]
                    tunnel: w455 -> [w460 w491]
                    frame True {
                      # "Ramp Up"
                      n178 = local read "First?"() -> (w471:bool)
                      n179 = case shown="False" w471 {
                        tunnel: [TRUE ("Save") FALSE ("Save")] -> w462
                        tunnel: [w483 w489] -> w465
                        frame False {
                          n180 = local read "Counter"() -> (w486:i8)
                          n181 = local write "Actual Polarization"(0.0 ("Actual Polarization")) -> ()
                          n182 = Increment(x=w486) -> (x+1=w483:i8)
                          n183 = local write "Counter"(w483) -> ()
                        }
                        frame True {
                          n184 = local read "Counter"() -> (w489:i8)
                          n185 = local write "First?"(FALSE ("First?")) -> ()
                        }
                      }
                      n186 = local write "Read?"(FALSE ("Read?")) -> ()
                      n187 = Number To Fractional String(number=w467, precision (6)=i16 3) -> (F-format string=w469:string)  [unwired: 2 in]
                      n188 = local read "Record ALL"() -> (w466:bool)
                      n189 = Concatenate Strings("SETP 1," ("write buffer"), w469) -> (w461:string)
                      n190 = case shown="True" w466 {
                        tunnel: w465 -> [_ w482]
                        tunnel: [FALSE w481] -> w463
                        frame False {
                        }
                        frame True {
                          n191 = local read "Max Countl"() -> (w480:i32)
                          n192 = Greater?(x=w482, y=w480) -> (0:w481:bool)
                        }
                      }
                      n193 = local write "Reset"(w462) -> ()
                      n194 = case shown="True" w463 {
                        tunnel: w461 -> [w476 _]
                        tunnel: w460 -> [w474 w477]
                        tunnel: [w473 w477] -> w459
                        frame False {
                          n195 = local read "Lake Shore"() -> (w475:refnum<visa-resource-name>)
                          n196 = VISA Write(VISA resource name=w475, write buffer=w476, error in (no error)=w474) -> (error out=w473:errorcluster)  [unwired: 2 out]
                        }
                        frame True {
                          n197 = local write "New"(TRUE ("New")) -> ()
                        }
                      }
                      "Up/Down 2" <- FALSE ("Up/Down")
                    }
                    frame False {
                      n198 = Equal?(x=w495, y=w492) -> (x = y?=w493:bool)
                      n199 = case shown="True" w493 {
                        tunnel: [w497 w501] -> w496
                        tunnel: w494 -> [_ w500]
                        tunnel: w491 -> [w497 w502]
                        frame False {
                        }
                        frame True {
                          w498 = TRUE ("Reset")
                          # "Ramp Dn"
                          n200 = local write "Up/Down 2"(w498) -> ()
                          n201 = Number To Fractional String(number=w500, precision (6)=i16 3) -> (F-format string=w504:string)  [unwired: 2 in]
                          n202 = local write "Reset"(w498) -> ()
                          n203 = local read "Lake Shore"() -> (w499:refnum<visa-resource-name>)
                          n204 = Concatenate Strings("SETP 1," ("write buffer"), w504) -> (w506:string)
                          n205 = VISA Write(VISA resource name=w499, write buffer=w506, error in (no error)=w502) -> (error out=w501:errorcluster)  [unwired: 2 out]
                        }
                      }
                      n206 = local write "Read?"(FALSE ("Read?")) -> ()
                    }
                  }
                }
              }
              n207 = local read "Magnet"() -> (w378:bool)
              n208 = case shown="False" w378 {
                tunnel: [Mode."StepDelta" ("Enum") Mode."Plot" ("Enum")] -> w380
                frame False {
                }
                frame True {
                }
              }
            }
            frame "StepDelta" {
              n209 = flat-sequence {
                tunnel: w508 -> [w524]
                tunnel: [w523] -> w507
                frame #0 {
                  # "Check if it is time to step Field"
                  n210 = local read "Sweep Rate (T/min)"() -> (w525:dbl)
                  n211 = local read "B/V (T/V)"() -> (w517:dbl)
                  n212 = local read "Time Lag"() -> (w521:dbl)
                  n213 = xnode "Sweep Delay"("SweepRate"=w525, "Resolution"=0.001 ("Voltage Step (V)"), "BpV"=w517) -> ("Result"=w522:dbl)  [unwired: 1 in, 1 out]
                  n214 = Divide(x=w521, y=w522) -> (x/y=w519:dbl)
                  n215 = Multiply(x=0.001 ("y"), y=w519) -> (x*y=w518:dbl)
                  "deltaUaux" <- w518
                  n216 = stacked-sequence {
                    tunnel: w524 -> [_ w549]
                    tunnel: [_ w548] -> w523
                    tunnel: w518 -> [w527 _]
                    frame #0 {
                      n217 = local read "Actual Voltage (V)"() -> (w532:dbl)
                      n218 = local read "Up/Down"() -> (w533:bool)
                      n219 = Add(x=w532, y=w527) -> (x+y=w529:dbl)
                      n220 = Subtract(x=w532, y=w527) -> (x-y=w528:dbl)
                      n221 = Select(t=w528, s=w533, f=w529) -> (s? t:f=w531:dbl)
                      "Actual Voltage (V)" <- w531
                      n222 = local read "V/I (Ohm)"() -> (w534:dbl)
                      n223 = local read "B/V (T/V)"() -> (w535:dbl)
                      n224 = xnode "AUXtoB"("BpV"=w535, "Rm"=w534, "Aux"=w531) -> ("Result"=w530:dbl)  [unwired: 1 in, 1 out]
                      n225 = local write "Actual Field (T)"(w530) -> ()
                    }
                    frame #1 {
                      n226 = local read "Actual Voltage (V)"() -> (w554:dbl)
                      n227 = local read "Lock_in_Amplifier"() -> (w550:refnum<visa-resource-name>)
                      n228 = Format Into String(w554) -> (resulting string=w553:string)  [unwired: 3 in, 1 out]
                      n229 = Concatenate Strings("AUXV 1,", w553) -> (w551:string)
                      n230 = VISA Write(VISA resource name=w550, write buffer=w551, error in (no error)=w549) -> (error out=w548:errorcluster)  [unwired: 2 out]
                    }
                  }
                }
              }
            }
            frame "Plot" {
              # "dI"
              n231 = local read "P(uC/mm^2)"() -> (w568:dbl[])
              n232 = local read "Actual Polarization"() -> (w567:dbl)
              n233 = local read "Actual Current (pA)"() -> (w569:dbl)
              n234 = local read "Time Lag"() -> (w581:dbl)
              n235 = Multiply(x=w569, y=w581) -> (x*y=w573:dbl)
              n236 = Divide(x=w573, y="Sample area (mm^2)") -> (x/y=w572:dbl)
              n237 = Add(x=w572, y=w567) -> (x+y=w571:dbl)
              "Actual Polarization" <- w571
              n238 = local read "Temp/Magnetic Field"() -> (w582:bool)
              n239 = Build Array (concatenate)(w568, w571) -> (→"P(uC/mm^2)":dbl[])
              n240 = case shown="False" w582 {
                tunnel: w579 -> [_ w642]
                tunnel: w576 -> [_ w624]
                tunnel: w571 -> [w589 w625]
                frame False {
                  # "Magnetic Field plotting"
                  n241 = local read "Up/Down"() -> (w594:bool)
                  n242 = case shown="True" w594 {
                    frame True {
                      # "Down"
                      n243 = local read "I(B) 3"() -> (w604:cluster{dbl[], dbl[]}[])
                      n244 = local read "I(B) 3"() -> (w608:cluster{dbl[], dbl[]}[])
                      n245 = Index Array(array=w604, index=1) -> (element=w602:cluster{dbl[], dbl[]})
                      n246 = Unbundle(w602) -> (w601:dbl[], w600:dbl[])
                      n247 = Index Array(array=w608, index=i8 0 ("t")) -> (element=w605:cluster{dbl[], dbl[]})
                      n248 = local read "Actual Current (pA)"() -> (w595:dbl)
                      n249 = local read "Actual B Field (T)"() -> (w597:dbl)
                      n250 = Build Array (concatenate)(w601, w597) -> (w599:dbl[])
                      n251 = Build Array (concatenate)(w600, w595) -> (w598:dbl[])
                      n252 = Bundle(w599, w598) -> (w596:cluster{dbl[], dbl[]})  [unwired: 1 in]
                      n253 = Build Array(w605, w596) -> (w606:cluster{dbl[], dbl[]}[])
                      n254 = local write "I(B) 3"(w606) -> ()
                    }
                    frame False {
                      # "Up"
                      n255 = local read "I(B) 3"() -> (w620:cluster{dbl[], dbl[]}[])
                      n256 = local read "I(B) 3"() -> (w622:cluster{dbl[], dbl[]}[])
                      n257 = Index Array(array=w620, index=0) -> (element=w618:cluster{dbl[], dbl[]})
                      n258 = Unbundle(w618) -> (w617:dbl[], w616:dbl[])
                      n259 = Index Array(array=w622, index=i8 1 ("t")) -> (element=w611:cluster{dbl[], dbl[]})
                      n260 = local read "Actual B Field (T)"() -> (w612:dbl)
                      n261 = Build Array (concatenate)(w617, w612) -> (w615:dbl[])
                      n262 = local read "Actual Current (pA)"() -> (w609:dbl)
                      n263 = Build Array (concatenate)(w616, w609) -> (w614:dbl[])
                      n264 = Bundle(w615, w614) -> (w613:cluster{dbl[], dbl[]})  [unwired: 1 in]
                      n265 = Build Array(w613, w611) -> (w610:cluster{dbl[], dbl[]}[])
                      n266 = local write "I(B) 3"(w610) -> ()
                    }
                  }
                  n267 = local read "Actual B Field (T)"() -> (w591:dbl)
                  n268 = local read "P(B)"() -> (w593:cluster{"yi":dbl[], dbl[]})
                  n269 = Unbundle(w593) -> ("yi"=w592:dbl[], w590:dbl[])
                  n270 = Build Array (concatenate)(w592, w591) -> (w588:dbl[])
                  n271 = Build Array (concatenate)(w590, w589) -> (w587:dbl[])
                  n272 = Bundle(w588, w587) -> (→"P(B)":cluster{dbl[], dbl[]})  [unwired: 1 in]
                }
                frame True {
                  # "Temperature plotting"
                  n273 = Quotient & Remainder(x=w642, y="Save Period") -> (x-y*floor(x/y)=w623:dbl)  [unwired: 1 out]
                  n274 = Greater?(x=w624, y=w623) -> (0:w640:bool)
                  n275 = local read "Actual Temperature (K)"() -> (w627:dbl)
                  n276 = local read "Actual Current (pA)"() -> (w633:dbl)
                  n277 = local read "P(T)"() -> (w629:cluster{"yi":dbl[], dbl[]})
                  n278 = local read "I(T)"() -> (w639:cluster{dbl[], dbl[]})
                  n279 = case shown="True" w640 {
                    frame False {
                    }
                    frame True {
                      n280 = local write "Reset"(TRUE) -> ()
                    }
                  }
                  n281 = Unbundle(w629) -> ("yi"=w630:dbl[], w626:dbl[])
                  n282 = Unbundle(w639) -> (w637:dbl[], w636:dbl[])
                  n283 = Build Array (concatenate)(w630, w627) -> (w631:dbl[])
                  n284 = Build Array (concatenate)(w626, w625) -> (w632:dbl[])
                  n285 = Build Array (concatenate)(w637, w627) -> (w635:dbl[])
                  n286 = Build Array (concatenate)(w636, w633) -> (w634:dbl[])
                  n287 = Bundle(w635, w634) -> (→"I(T)":cluster{dbl[], dbl[]})  [unwired: 1 in]
                  n288 = Bundle(w631, w632) -> (→"P(T)":cluster{dbl[], dbl[]})  [unwired: 1 in]
                }
              }
            }
            frame "Save" {
              n289 = local read "Reset"() -> (w644:bool)
              n290 = case shown="True" w644 {
                tunnel: w649 -> [w666 w668]
                tunnel: [w666 w671] -> w654
                tunnel: w648 -> [w665 w669]
                tunnel: [w665 w671] -> w653
                tunnel: w650 -> [w664 w670]
                tunnel: [w664 w671] -> w652
                tunnel: [w663 w671] -> w651
                tunnel: w647 -> [w663 w667]
                frame False {
                }
                frame True {
                  n291 = stacked-sequence {
                    tunnel: [_ _ w751] -> w671
                    tunnel: w670 -> [_ w746 _]
                    tunnel: w669 -> [w674 w744 _]
                    tunnel: w668 -> [w675 w745 _]
                    tunnel: w667 -> [w673 w742 _]
                    frame #0 {
                      n292 = local read "Temp/Magnetic Field"() -> (w672:bool)
                      n293 = case shown="True" w672 {
                        tunnel: w675 -> [w702 w729]
                        tunnel: w674 -> [w701 w728]
                        tunnel: w673 -> [w692 w719]
                        frame False {
                          n294 = local read "B array"() -> (w686:dbl[])
                          n295 = local read "Counter"() -> (w700:i8)
                          n296 = local read "Averaged I(B)"() -> (w677:dbl[][])
                          n297 = local read "Up/Down"() -> (w703:bool)
                          n298 = local read "Sample area (mm^2)"() -> (w682:dbl)
                          n299 = call "Average_IBP_curves_baseline.vi"("I in"=w701, "Averaged P(B) In"="Averaged P(B)", "Counter"=w700, "B0"="Threshold B (T)", "Averaged I(B) In"=w677, "t in"=w692, "B in"=w702, "Averaged dt in"="Averaged dt", "Up/Down"=w703, "Sample area(mm^2)"=w682, "B array"=w686) -> ("Averaged dt Out"=w689:dbl[][], "Averaged P(B) Out"=w678:dbl[][], "BaselineSubtracted I(B)"=w676:dbl[][])  [unwired: 1 in, 1 out]
                          "Averaged I(B)" <- w676
                          n300 = Index Array(array=w678, index (row)=0 ("disabled index (col)")) -> (element=w687:dbl[])  [unwired: 1 in]
                          n301 = Index Array(array=w678, index (row)=1 ("disabled index (col)")) -> (element=w688:dbl[])  [unwired: 1 in]
                          n302 = Index Array(array=w676, index (row)=0 ("disabled index (col)")) -> (element=w694:dbl[])  [unwired: 1 in]
                          n303 = Index Array(array=w676, index (row)=1 ("disabled index (col)")) -> (element=w693:dbl[])  [unwired: 1 in]
                          n304 = local write "Averaged dt"(w689) -> ()
                          n305 = Bundle("B array"=w686, "Averaged P(B) Out"=w687) -> (w685:T7)  [unwired: 1 in]
                          n306 = Bundle("B array"=w686, "Averaged P(B) Out"=w688) -> (w684:T7)  [unwired: 1 in]
                          n307 = local write "Averaged P(B)"(w678) -> ()
                          n308 = Bundle("B array"=w686, "BaselineSubtracted I(B)"=w694) -> (w699:T8)  [unwired: 1 in]
                          n309 = Bundle("B array"=w686, "BaselineSubtracted I(B)"=w693) -> (w698:T8)  [unwired: 1 in]
                          n310 = Build Array(w685, w684) -> (→"P(B) /Averaged/":T9)
                          n311 = Build Array(w699, w698) -> (→"I(B) /Averaged/":T10)
                        }
                        frame True {
                          n312 = local read "T array"() -> (w714:dbl[])
                          n313 = local read "Counter"() -> (w727:i8)
                          n314 = local read "Averaged I(T)"() -> (w706:dbl[][])
                          n315 = local read "Up/Down"() -> (w730:bool)
                          n316 = local read "Averaged dt"() -> (w705:dbl[][])
                          n317 = local read "Sample area (mm^2)"() -> (w710:dbl)
                          n318 = call "Average_ITP_curves.vi"("I in"=w728, "Averaged P(T) In"="Averaged P(T)", "Counter"=w727, "Averaged I(T) In"=w706, "t in"=w719, "T in"=w729, "Averaged dt in"=w705, "Up/Down"=w730, "Sample area(mm^2)"=w710, "T array"=w714) -> ("Averaged I(B) out"=w704:dbl[][], "Averaged dt Out"=w717:dbl[][], "Averaged P(T) Out"=w707:dbl[][])  [unwired: 3 in]
                          "Averaged I(T)" <- w704
                          n319 = Index Array(array=w707, index (row)=0 ("disabled index (col)")) -> (element=w715:dbl[])  [unwired: 1 in]
                          n320 = Index Array(array=w707, index (row)=1 ("disabled index (col)")) -> (element=w716:dbl[])  [unwired: 1 in]
                          n321 = Index Array(array=w704, index (row)=0 ("disabled index (col)")) -> (element=w721:dbl[])  [unwired: 1 in]
                          n322 = Index Array(array=w704, index (row)=1 ("disabled index (col)")) -> (element=w720:dbl[])  [unwired: 1 in]
                          n323 = local write "Averaged dt"(w717) -> ()
                          n324 = Bundle("T array"=w714, "Averaged P(T) Out"=w715) -> (w713:T11)  [unwired: 1 in]
                          n325 = Bundle("T array"=w714, "Averaged P(T) Out"=w716) -> (w712:T11)  [unwired: 1 in]
                          n326 = local write "Averaged P(T)"(w707) -> ()
                          n327 = Bundle("T array"=w714, "Averaged I(B) out"=w721) -> (w726:T12)  [unwired: 1 in]
                          n328 = Bundle("T array"=w714, "Averaged I(B) out"=w720) -> (w725:T12)  [unwired: 1 in]
                          n329 = Build Array(w713, w712) -> (→"P(T) /Averaged/":T13)
                          n330 = Build Array(w726, w725) -> (→"I(T) /Averaged/":T14)
                        }
                      }
                    }
                    frame #1 {
                      # "Save and Reset"
                      n331 = local read "Measurement File"() -> (w737:path)
                      n332 = local read "Up/Down"() -> (w732:bool)
                      n333 = local read "P(uC/mm^2)"() -> (w743:dbl[])
                      n334 = case shown="False" w732 {
                        tunnel: [w748 w749] -> w731
                        frame False {
                          n335 = local read "Measurement File_dn"() -> (w748:path)
                        }
                        frame True {
                          n336 = local read "Measurement File_up"() -> (w749:path)
                        }
                      }
                      n337 = Build Array(w746, w745, w744, w742, w743) -> (w736:dbl[][])
                      n338 = case shown="True" "Reset IB?" {
                        frame False {
                        }
                        frame True {
                          n339 = local read "Up/Down"() -> (w750:bool)
                          n340 = case shown="False" w750 {
                            frame False {
                              n341 = invoke on="I(B) 3" class="XYGraph (strict)" method="Reinit To Default"() -> ()  [unwired: 3 in, 3 out]
                              n342 = invoke on="I(T)" class="XYGraph (strict)" method="Reinit To Default"() -> ()  [unwired: 3 in, 3 out]
                            }
                            frame True {
                            }
                          }
                        }
                      }
                      n343 = call-poly <vilib>:"Write Delimited Spreadsheet.vi"("file path (dialog if empty)"=w737, "format (%.3f)"="%.5g", "2D data"=w736, "append to file? (F)"=TRUE, "transpose? (F)"=TRUE) -> ()  [unwired: 9 in, 2 out]
                      n344 = call-poly <vilib>:"Write Delimited Spreadsheet.vi"("file path (dialog if empty)"=w731, "format (%.3f)"="%.5g", "2D data"=w736, "append to file? (F)"=TRUE ("transpose? (F)"), "transpose? (F)"=FALSE ("append to file? (F)")) -> ()  [unwired: 9 in, 2 out]
                      n345 = local write "Reset"(FALSE ("Save")) -> ()
                    }
                    frame #2 {
                      w751 = dbl[] []
                      n346 = local write "P(uC/mm^2)"(w751) -> ()
                    }
                  }
                }
              }
              n347 = local read "New"() -> (w646:bool)
              n348 = case shown="False" w646 {
                tunnel: [Mode."Return" ("Enum") Mode."New" ("Enum")] -> w658
                tunnel: [TRUE FALSE] -> w645
                frame False {
                }
                frame True {
                }
              }
            }
            frame "New" {
              n349 = stacked-sequence {
                seq-local: [_ _ _ _ w853 _ _] -> [_ _ _ _ _ w862 _]
                seq-local: [_ _ w807 _ _ _ _] -> [_ _ _ _ w852 _ _]
                tunnel: T6 {"Com Port"=1, "ISOBUS Address"=0, "GPIB Address"=25, "Communication"=enum."GPIB"} ("Address") -> [_ _ w806 w847 _ _ _]
                tunnel: w754 -> [_ _ w808 _ _ w863 _]
                tunnel: [_ _ _ _ _ w865 _] -> w753
                tunnel: w752 -> [_ w787 _ _ _ _ _]
                frame #0 {
                  w780 = 1 ("index (row)")
                  w779 = 0 ("index (row)")
                  # "Save averages"
                  n350 = local read "Measurement File_average"() -> (w767:path)
                  n351 = local read "Averaged P(B)"() -> (w778:dbl[][])
                  n352 = local read "Averaged dt"() -> (w776:dbl[][])
                  n353 = local read "I(B) /Averaged/"() -> (w768:cluster{"B array":dbl[], dbl[]}[])
                  n354 = Index Array(array=w776, index (row)=w779) -> (element=w777:dbl[])  [unwired: 1 in]
                  n355 = Index Array(array=w776, index (row)=w780) -> (element=w784:dbl[])  [unwired: 1 in]
                  n356 = Index Array(array=w768, index=1) -> (element=w772:cluster{"B array":dbl[], dbl[]})
                  n357 = Index Array(array=w768, index=0) -> (element=w771:cluster{"B array":dbl[], dbl[]})
                  n358 = Unbundle(w772) -> ("B array"=w782:dbl[], w783:dbl[])
                  n359 = Unbundle(w771) -> ("B array"=w773:dbl[], w774:dbl[])
                  n360 = Index Array(array=w778, index (row)=w779) -> (element=w781:dbl[])  [unwired: 1 in]
                  n361 = Index Array(array=w778, index (row)=w780) -> (element=w785:dbl[])  [unwired: 1 in]
                  n362 = Build Array(w773, w774, w777, w781, w782, w783, w784, w785) -> (w775:dbl[][])
                  n363 = call-poly <vilib>:"Write Delimited Spreadsheet.vi"("file path (dialog if empty)"=w767, "format (%.3f)"="%.5g", "2D data"=w775, "append to file? (F)"=TRUE ("transpose? (F)"), "transpose? (F)"=TRUE ("append to file? (F)")) -> ()  [unwired: 9 in, 2 out]
                }
                frame #1 {
                  w793 = dbl[] []
                  w802 = dbl[] []
                  # "Reset Flags"
                  n364 = Get Date/Time In Seconds() -> (seconds since 1Jan1904=w803:timestamp)
                  n365 = local write "Up/Down"(TRUE ("Up/Down")) -> ()
                  n366 = local write "First?"(TRUE ("First?")) -> ()
                  n367 = local write "Offset?"(FALSE ("Offset?")) -> ()
                  n368 = local write "New"(FALSE ("New")) -> ()
                  n369 = local write "P(uC/mm^2)"(w802) -> ()
                  n370 = local write "Start time"(w803) -> ()
                  n371 = local write "Offset array"(w802) -> ()
                  n372 = local write "Actual Polarization"(0.0 ("Actual Polarization")) -> ()
                  n373 = local write "Up/Down"(TRUE ("Up/Down")) -> ()
                  n374 = local write "Reset"(FALSE ("Reset")) -> ()
                  n375 = local read "B array"() -> (w796:dbl[])
                  n376 = local write "Counter"(i8 0 ("Counter")) -> ()
                  n377 = invoke on="P(B)" class="XYGraph (strict)" method="Reinit To Default"() -> ()  [unwired: 3 in, 3 out]
                  n378 = invoke on="I(B) 3" class="XYGraph (strict)" method="Reinit To Default"() -> ()  [unwired: 3 in, 3 out]
                  n379 = Multiply(x=w796, y=0.0) -> (x*y=w797:dbl[])
                  n380 = Build Array(w793, w793) -> (w801:dbl[][])
                  n381 = Bundle("B array"=w796, w797) -> (w798:cluster{"B array":dbl[], dbl[]})  [unwired: 1 in]
                  n382 = local write "Averaged I(B)"(w801) -> ()
                  n383 = Build Array(w798, w798) -> (w799:cluster{"B array":dbl[], dbl[]}[])
                  n384 = local write "I(B) /Averaged/"(w799) -> ()
                  n385 = local write "Measuring"(FALSE ("Measuring")) -> ()
                  n386 = Flush Queue(queue=w787) -> (remaining elements=→"remaining elements 2":T1)  [unwired: 1 in, 2 out]
                }
                frame #2 {
                  # "Step"
                  n387 = local read "Sweep Rate Array"() -> (w812:dbl[])
                  n388 = local read "j"() -> (w813:i32)
                  n389 = Increment(x=w813) -> (x+1=w809:i32)
                  n390 = Array Size(array=w812) -> (size(s)=w811:i32)
                  n391 = Less?(x=w809, y=w811) -> (x < y?=w810:bool)
                  "Step Rate" <- w810
                  n392 = case shown="True" w810 {
                    tunnel: w809 -> [_ w840]
                    tunnel: w808 -> [w816 w839]
                    tunnel: [w815 w839] -> w807
                    tunnel: w806 -> [w814 _]
                    frame False {
                      # "Step Temp?"
                      n393 = local read "Temperature Array"() -> (w820:dbl[])
                      n394 = local read "i"() -> (w821:i32)
                      n395 = Increment(x=w821) -> (x+1=w818:i32)
                      n396 = local write "j"(0 ("f")) -> ()
                      n397 = Array Size(array=w820) -> (size(s)=w819:i32)
                      n398 = Less?(x=w818, y=w819) -> (x < y?=w817:bool)
                      "Step Temp" <- w817
                      n399 = case shown="False" w817 {
                        tunnel: w818 -> [_ w838]
                        tunnel: w816 -> [w826 w837]
                        tunnel: [w825 w837] -> w815
                        tunnel: w814 -> [w824 _]
                        frame False {
                          # "Heater OFF"
                          # "Finished"
                          n400 = local write "i"(0 ("i")) -> ()
                          n401 = stacked-sequence {
                            tunnel: w826 -> [w830 _ _]
                            tunnel: [w829 _ _] -> w825
                            tunnel: w824 -> [_ w834 w835]
                            frame #0 {
                              n402 = local read "Lake Shore"() -> (w831:refnum<visa-resource-name>)
                              n403 = VISA Write(VISA resource name=w831, write buffer="RANGE,1,0", error in (no error)=w830) -> (error out=w829:errorcluster)  [unwired: 2 out]
                            }
                            frame #1 {
                              n404 = call "ips_switchHeaterOff.vi"("Instrument address"=w834, "Rate"=2.0) -> ()  [unwired: 1 out]
                            }
                            frame #2 {
                              n405 = call "GPIB - BusCommand.vi"("Command"="H0", "Address"=w835) -> ()  [unwired: 2 out]
                            }
                          }
                          n406 = local write "Record ALL"(FALSE ("Record ALL")) -> ()
                          "Finished" <- TRUE
                        }
                        frame True {
                          n407 = local write "i"(w838) -> ()
                        }
                      }
                    }
                    frame True {
                      n408 = local write "j"(w840) -> ()
                    }
                  }
                }
                frame #3 {
                  # "Set rates"
                  n409 = local read "Sweep Rate Array"() -> (w846:dbl[])
                  n410 = local read "j"() -> (w845:i32)
                  n411 = local read "j"() -> (w843:i32)
                  n412 = Index Array(array=w846, index=w845) -> (element=w844:dbl)
                  n413 = Number To Fractional String(number=w844, precision (6)=i16 3) -> (F-format string=w850:string)  [unwired: 2 in]
                  n414 = Index Array(array="Max count array", index=w843) -> (element=w841:i32)
                  n415 = local write "Max Countl"(w841) -> ()
                  n416 = Concatenate Strings("T" ("format string"), w850) -> (w851:string)
                  n417 = call "GPIB - BusCommand.vi"("Command"=w851, "Address"=w847) -> ()  [unwired: 2 out]
                  n418 = local write "Sweep Rate (T/min)"(w844) -> ()
                }
                frame #4 {
                  # "Set temperature"
                  n419 = local read "Temperature Array"() -> (w856:dbl[])
                  n420 = local read "i"() -> (w855:i32)
                  n421 = Index Array(array=w856, index=w855) -> (element=w854:dbl)
                  n422 = local read "Lake Shore"() -> (w858:refnum<visa-resource-name>)
                  n423 = Number To Fractional String(number=w854, precision (6)=i16 3) -> (F-format string=w859:string)  [unwired: 2 in]
                  n424 = Concatenate Strings("SETP 1," ("write buffer"), w859) -> (w861:string)
                  n425 = VISA Write(VISA resource name=w858, write buffer=w861, error in (no error)=w852) -> (error out=w853:errorcluster)  [unwired: 2 out]
                }
                frame #5 {
                  n426 = local read "Finished"() -> (w864:bool)
                  n427 = case shown="False" w864 {
                    tunnel: [w878 w915] -> w865
                    tunnel: w863 -> [_ _]
                    tunnel: w862 -> [w875 w915]
                    frame False {
                      w873 = "_" ("string")
                      # "Wait, create Files"
                      n428 = local read "Temperature Array"() -> (w905:dbl[])
                      n429 = local read "Sweep Rate Array"() -> (w901:dbl[])
                      n430 = local read "i"() -> (w904:i32)
                      n431 = local read "j"() -> (w902:i32)
                      n432 = Index Array(array=w905, index=w904) -> (element=w903:dbl)
                      n433 = Index Array(array=w901, index=w902) -> (element=w870:dbl)
                      n434 = Round Toward -Infinity(1:w870) -> (0:w871:dbl)
                      n435 = Number To Fractional String(use system decimal point (T)=TRUE, number=w903, precision (6)=i16 1) -> (F-format string=w906:string)  [unwired: 1 in]
                      n436 = Subtract(x=w870, y=w871) -> (x-y=w872:dbl)
                      n437 = Equal To 0?(x=w872) -> (x = 0?=w869:bool)
                      n438 = Select(t=i16 0 ("precision (6)"), s=w869, f=i16 2 ("precision (6)")) -> (s? t:f=w866:i16)
                      n439 = Number To Fractional String(use system decimal point (T)=TRUE, number=w870, precision (6)=w866) -> (F-format string=w874:string)  [unwired: 1 in]
                      n440 = Concatenate Strings("Directory", "\\" ("string"), "FileName", w873, w906, "K" ("string"), w873, w874, "Tpm" ("string")) -> (w895:string)
                      n441 = Search and Replace String(replace all?=TRUE ("replace all? (F)"), input string=w895, search string=".", replace string="p" ("substring (\"\")"), error in=w875) -> (result string=w890:string, error out=w885:errorcluster)  [unwired: 3 in, 2 out]
                      n442 = local write "Step Rate"(FALSE ("Step Rate")) -> ()
                      n443 = Concatenate Strings(w890, ".txt" ("string")) -> (w889:string)
                      n444 = local read "Step Temp"() -> (w879:bool)
                      n445 = String To Path(string=w889) -> (path=w888:path)
                      n446 = Open/Create/Replace File(file path (use dialog)=w888, error in=w885, operation (0:open)=T5."open or create") -> (refnum out=w877:refnum<file>, error out=w878:errorcluster)  [unwired: 3 in, 1 out]
                      n447 = local write "refnum out"(w877) -> ()
                      n448 = Refnum to Path(1:w877) -> (0:w880:path)
                      n449 = call "Create_sweep_files.vi"("Measurement File"=w880) -> ("Path 3"=w883:path, "Path 2"=w882:path, "Path"=w881:path)  [unwired: 8 in]
                      n450 = local write "Measurement File"(w880) -> ()
                      n451 = case shown="True" w879 {
                        frame False {
                        }
                        frame True {
                          n452 = Get Date/Time In Seconds() -> (seconds since 1Jan1904=w908:timestamp)
                          n453 = local write "Step Temp"(FALSE ("Step Temp")) -> ()
                          n454 = while {
                            tunnel: w908 -> [w913]
                            stop <- w910 stop-if-true
                            n455 = Get Date/Time In Seconds() -> (seconds since 1Jan1904=w914:timestamp)
                            n456 = Subtract(x=w914, y=w913) -> (x-y=w912:dbl)
                            "Wait (s)" <- w912
                            n457 = Greater Or Equal?(x=w912, y="secs to wait") -> (x >= y?=w910:bool)
                          }
                        }
                      }
                      n458 = local write "Measurement File_dn"(w883) -> ()
                      n459 = local write "Measurement File_average"(w881) -> ()
                      n460 = local write "Measurement File_up"(w882) -> ()
                    }
                    frame True {
                    }
                  }
                }
                frame #6 {
                  n461 = local read "Finished"() -> (w916:bool)
                  n462 = case shown="True" w916 {
                    frame False {
                      n463 = local write "Measuring"(TRUE ("Measuring")) -> ()
                    }
                    frame True {
                      n464 = local write "Measure /Pause"(FALSE ("Measure /Pause")) -> ()
                    }
                  }
                }
              }
            }
            frame "Return" {
            }
          }
        }
      }
      frame Error {
        # "Return true for any case which should stop the loop."
      }
    }
  }
  n465 = VISA Read(VISA resource name=w10, byte count=u32 100, error in (no error)=w12) -> (VISA resource name out=w9:refnum<visa-resource-name>, read buffer=w8:string, error out=w11:errorcluster)  [unwired: 1 out]
  n466 = VISA Open(error in (no error)=w11, VISA resource name="Magnetic Field") -> (VISA resource name=w105:refnum<visa-resource-name>, error out=w87:errorcluster)  [unwired: 3 in]
  n467 = VISA Open(error in (no error)=w87, VISA resource name="Lake Shore") -> (VISA resource name=w82:refnum<visa-resource-name>, error out=w51:errorcluster)  [unwired: 3 in]
  n468 = VISA Write(VISA resource name="Lake Shore", write buffer="KRDG?a", error in (no error)=w51) -> (VISA resource name out=w48:refnum<visa-resource-name>, error out=w47:errorcluster)  [unwired: 1 out]
  n469 = VISA Read(VISA resource name=w48, byte count=w54, error in (no error)=w47) -> (VISA resource name out=w45:refnum<visa-resource-name>, read buffer=w59:string, error out=w46:errorcluster)  [unwired: 1 out]
  n470 = VISA Write(VISA resource name=w45, write buffer="SETP?a", error in (no error)=w46) -> (VISA resource name out=w44:refnum<visa-resource-name>, error out=w43:errorcluster)  [unwired: 1 out]
  n471 = VISA Read(VISA resource name=w44, byte count=w54, error in (no error)=w43) -> (VISA resource name out=w41:refnum<visa-resource-name>, read buffer=w58:string, error out=w42:errorcluster)  [unwired: 1 out]
  n472 = VISA Write(VISA resource name=w41, write buffer="RANGE?a", error in (no error)=w42) -> (VISA resource name out=w39:refnum<visa-resource-name>, error out=w40:errorcluster)  [unwired: 1 out]
  n473 = Fract/Exp String To Number(string=w59) -> (number=w57:dbl)  [unwired: 3 in, 1 out]
  n474 = VISA Read(VISA resource name=w39, byte count=w54, error in (no error)=w40) -> (read buffer=w53:string, error out=w50:errorcluster)  [unwired: 2 out]
  n475 = Fract/Exp String To Number(string=w58) -> (number=w56:dbl)  [unwired: 3 in, 1 out]
  n476 = Fract/Exp String To Number(string=w53) -> (number=w49:dbl)  [unwired: 3 in, 1 out]
  n477 = local write "Actual Temperature (K)"(w57) -> ()
  n478 = local write "Setpoint Temperature (K)"(w56) -> ()
  n479 = local write "Heater Range"(w49) -> ()
  n480 = case shown="True" w64 {
    frame False {
    }
    frame True {
      n481 = invoke on="P(T)" class="XYGraph (strict)" method="Reinit To Default"() -> ()  [unwired: 3 in, 3 out]
      n482 = invoke on="I(T)" class="XYGraph (strict)" method="Reinit To Default"() -> ()  [unwired: 3 in, 3 out]
    }
  }
  n483 = Decimal String To Number(string=w8) -> (number=w7:i32)  [unwired: 2 in, 1 out]
  n484 = local write "Keithley (IV conv) averaging"(w7) -> ()
  n485 = while {
    shift-right: [w947] -> w103
    shift-left: w84 -> [w948]
    shift-right: [w949] -> w108
    shift-left: w109 -> [w950]
    tunnel: w9 -> [w946]
    tunnel: w105 -> [w945]
    tunnel: w50 -> [_]
    tunnel: [w939] -> _
    tunnel: w92 -> [w938]
    tunnel: w82 -> [w937]
    tunnel: w17 -> [w936]
    stop <- "stop" stop-if-true
    n486 = event shown="[7] \"Stop\": Value Change" {
      selector: _ -> [_ _ _ _ _ _ _ _ _ _ _ _ _ _ _ _]
      dyn-events: _ -> [_ _ _ _ _ _ _ _ _ _ _ _ _ _ _ _]
      timeout: 10 -> [_ _ _ _ _ _ _ _ _ _ _ _ _ _ _ _]
      tunnel: w950 -> [w960 w1006 w1024 w1034 w1048 w1119 w1123 w1127 w1167 w1183 w1200 w1243 w1260 w1276 w1286 w1297]
      tunnel: [w959 w1006 w1024 w1034 w1048 w1119 w1123 w1127 w1167 w1183 w1200 w1243 w1260 w1276 w1286 w1297] -> w949
      tunnel: w948 -> [w958 w1015 w1023 w1033 w1046 w1118 w1125 w1129 w1168 w1182 w1199 w1244 w1262 w1280 w1290 w1299]
      tunnel: [w957 w1007 w1023 w1033 w1045 w1120 w1125 w1128 _ w1182 w1199 w1244 w1261 w1279 w1289 w1298] -> w947
      tunnel: w946 -> [w956 w1016 _ _ _ _ _ _ _ _ _ _ _ _ _ _]
      tunnel: w945 -> [w955 _ _ _ _ _ _ _ _ _ _ _ _ _ _ _]
      tunnel: [w953 w1005 w1022 w1032 w1047 w1121 w1124 w1126 w1166 w1181 w1198 w1242 w1259 w1277 w1287 _] -> w939
      tunnel: w938 -> [w953 w1005 w1022 w1035 w1047 w1121 w1124 w1126 w1166 w1181 w1198 w1242 w1259 w1277 w1287 _]
      tunnel: w937 -> [_ _ _ _ _ _ _ _ _ _ _ _ w1263 w1278 w1291 w1296]
      tunnel: [_ _ _ _ _ _ _ _ w1168 _ _ _ _ _ _ _] -> _
      tunnel: w936 -> [w952 _ _ _ _ _ _ _ _ _ _ _ _ _ _ _]
      event Timeout {
        n487 = event-data() -> ()  [unwired: 1 in, 3 out]
        n488 = case shown="True" "Measuring" {
          tunnel: w960 -> [w962 w985]
          tunnel: [w962 w984] -> w959
          tunnel: w958 -> [w961 w963]
          tunnel: [w961 w983] -> w957
          tunnel: w956 -> [_ w976]
          tunnel: w955 -> [_ w975]
          tunnel: w952 -> [_ w966]
          frame False {
          }
          frame True {
            w974 = ":FETCh? " ("data")
            w977 = u32 1000 ("byte count")
            # "Generate the data here."
            n489 = case shown="No Error" w963 {
              selector: w963 -> [w997 w998]
              tunnel: [w997 w998] -> w971
              tunnel: [w996 _] -> w970
              frame No Error {
                n490 = Get Date/Time In Seconds() -> (seconds since 1Jan1904=w996:timestamp)
              }
              frame Error {
              }
            }
            n491 = VISA Write(VISA resource name=w976, write buffer=w974, error in (no error)=w971) -> (VISA resource name out=w982:refnum<visa-resource-name>, error out=w980:errorcluster)  [unwired: 1 out]
            n492 = VISA Write(VISA resource name=w975, write buffer=w974, error in (no error)=w980) -> (VISA resource name out=w981:refnum<visa-resource-name>, error out=w979:errorcluster)  [unwired: 1 out]
            n493 = VISA Read(VISA resource name=w982, byte count=w977, error in (no error)=w979) -> (read buffer=w972:string, error out=w978:errorcluster)  [unwired: 2 out]
            n494 = VISA Read(VISA resource name=w981, byte count=w977, error in (no error)=w978) -> (read buffer=w973:string, error out=w968:errorcluster)  [unwired: 2 out]
            n495 = case shown="True" "DaQ" {
              tunnel: w968 -> [w987 w993]
              tunnel: [w987 w992] -> w967
              tunnel: w966 -> [_ w991]
              tunnel: [0.0 ("Output") w989] -> w964
              frame False {
              }
              frame True {
                n496 = local read "Number of Samples"() -> (w995:i32)
                n497 = call-poly <vilib>:"DAQmx Read.vi"("task/channels in"=w991, "number of samples per channel"=w995, "error in"=w993) -> ("data"=w994:dbl[], "error out"=w992:errorcluster)  [unwired: 10 in, 1 out]
                n498 = call-poly <vilib>:"Mean.vi"("X"=w994) -> ("mean"=w990:dbl)  [unwired: 1 out]
                "Actual mean" <- w990
                n499 = call "N Point Running Average.vi"("n"="Moving average", "Input"=w990) -> ("Output"=w989:dbl)
              }
            }
            n500 = Bundle("seconds since 1Jan1904"=w970, "read buffer"=w972, "read buffer"=w973, "Output"=w964) -> (w969:T4)  [unwired: 1 in]
            n501 = Enqueue Element(queue=w985, element=w969, error in (no error)=w967) -> (queue out=w984:refnum<queue>, error out=w983:errorcluster)  [unwired: 1 in, 1 out]
          }
        }
      }
      event "Keithley (IV conv) averaging": Value Change {
        n502 = event-data() -> ()  [unwired: 1 in, 6 out]
        n503 = Number To Decimal String(number="Keithley (IV conv) averaging") -> (decimal integer string=w1013:string)  [unwired: 1 in]
        n504 = Concatenate Strings("VOLTage:DC:AVERage:COUNt " ("write buffer"), w1013) -> (w1012:string)
        n505 = VISA Write(VISA resource name=w1016, write buffer=w1012, error in (no error)=w1015) -> (VISA resource name out=w1011:refnum<visa-resource-name>, error out=w1009:errorcluster)  [unwired: 1 out]
        n506 = VISA Write(VISA resource name=w1011, write buffer="VOLTage:DC:AVERage:COUNt?", error in (no error)=w1009) -> (VISA resource name out=w1004:refnum<visa-resource-name>, error out=w1008:errorcluster)  [unwired: 1 out]
        n507 = VISA Read(VISA resource name=w1004, byte count=u32 100, error in (no error)=w1008) -> (read buffer=w1002:string, error out=w1007:errorcluster)  [unwired: 2 out]
        n508 = Decimal String To Number(string=w1002) -> (number=w1001:i32)  [unwired: 2 in, 1 out]
        n509 = Equal?(x="Keithley (IV conv) averaging", y=w1001) -> (x = y?=→"Confirm":bool)
      }
      event "Max Field (T)": Value Change {
        n510 = event-data() -> ()  [unwired: 1 in, 6 out]
        n511 = Divide(x="Max Field (T)", y="dB (T)") -> (x/y=w1019:dbl)
        n512 = for {
          N: w1019 -> [_]
          tunnel: "dB (T)" -> [w1029]
          tunnel: [w1026] -> w1018 mode=indexing
          tunnel: "Min Field (T)" -> [w1027]
          tunnel: [0.0] -> _ mode=indexing
          i -> [w1030]
          n513 = Multiply(x=w1030, y=w1029) -> (x*y=w1028:dbl)
          n514 = Add(x=w1028, y=w1027) -> (x+y=w1026:dbl)
        }
        "B array" <- w1018
      }
      event "Sweep Rate (T/min)": Value Change {
        n515 = event-data() -> ("NewVal"=w1036:dbl)  [unwired: 1 in, 5 out]
        n516 = local read "Magnet"() -> (w1031:bool)
        n517 = case shown="False" w1031 {
          tunnel: w1036 -> [_ w1043]
          tunnel: w1035 -> [w1037 w1039]
          tunnel: [w1037 w1038] -> w1032
          frame False {
          }
          frame True {
            n518 = Number To Fractional String(number=w1043, precision (6)=i16 3) -> (F-format string=w1041:string)  [unwired: 2 in]
            n519 = Concatenate Strings("T" ("format string"), w1041) -> (w1040:string)
            n520 = call "GPIB - BusCommand.vi"("Command"=w1040, "Address"=w1039) -> ("Address(thru)"=w1038:T6)  [unwired: 1 out]
          }
        }
      }
      event "Field To Zero": Value Change {
        n521 = event-data() -> ()  [unwired: 1 in, 6 out]
        n522 = Two Button Dialog(message="Do you want to switch off the field?", 1:"No" ("F button name (\"Cancel\")"), 2:"Yes" ("T button name (\"OK\")")) -> (T button?=w1052:bool)
        n523 = case shown="True" w1052 {
          tunnel: w1047 -> [_ w1057]
          tunnel: w1046 -> [w1053 w1055]
          tunnel: [w1053 w1054] -> w1045
          frame False {
          }
          frame True {
            n524 = local read "Magnet"() -> (w1056:bool)
            n525 = case shown="False" w1056 {
              tunnel: w1057 -> [_ w1109]
              tunnel: w1055 -> [w1060 w1106]
              tunnel: [w1059 w1106] -> w1054
              frame False {
                n526 = local read "Lock_in_Amplifier"() -> (w1058:refnum<visa-resource-name>)
                n527 = stacked-sequence {
                  seq-local: [w1063 _] -> [_ w1075]
                  seq-local: [w1061 _] -> [_ w1072]
                  tunnel: w1060 -> [w1065 _]
                  tunnel: [_ w1078] -> w1059
                  tunnel: w1058 -> [w1062 w1073]
                  frame #0 {
                    n528 = VISA Write(VISA resource name=w1062, write buffer="AUXV?1", error in (no error)=w1065) -> (VISA resource name out=w1069:refnum<visa-resource-name>, error out=w1064:errorcluster)  [unwired: 1 out]
                    n529 = VISA Read(VISA resource name=w1069, byte count=u32 1000, error in (no error)=w1064) -> (read buffer=w1066:string, error out=w1063:errorcluster)  [unwired: 2 out]
                    n530 = Fract/Exp String To Number(string=w1066) -> (number=w1061:dbl)  [unwired: 3 in, 1 out]
                  }
                  frame #1 {
                    w1081 = 0.001 ("Voltage Step (V)")
                    n531 = local read "Sweep Rate (T/min)"() -> (w1080:dbl)
                    n532 = local read "V/I (Ohm)"() -> (w1077:dbl)
                    n533 = local read "B/V (T/V)"() -> (w1071:dbl)
                    n534 = xnode "Sweep Delay"("SweepRate"=w1080, "Resolution"=w1081, "BpV"=w1071) -> ("Result"=w1079:dbl)  [unwired: 1 in, 1 out]
                    n535 = call "Universal_Ramping.vi"("milliseconds to wait"=w1079, "Initial Voltage (V)"=w1072, "error in (no error)"=w1075, "Voltage Step (V)"=w1081, "Final Voltage (V)"=0.0, "VISA resource name"=w1073) -> ("error out"=w1078:errorcluster, "Actual Voltage (V)"=w1070:dbl)  [unwired: 3 in, 1 out]
                    n536 = local write "Actual Voltage (V)"(w1070) -> ()
                    n537 = xnode "AUXtoB"("BpV"=w1071, "Rm"=w1077, "Aux"=w1070) -> ("Result"=w1076:dbl)  [unwired: 1 in, 1 out]
                    n538 = local write "Actual B Field (T)"(w1076) -> ()
                  }
                }
              }
              frame True {
                n539 = local read "Sweep Rate (T/min)"() -> (w1108:dbl)
                n540 = call "ips_switchHeaterOff.vi"("Instrument address"=w1109, "Rate"=w1108) -> ("B"=w1107:dbl)
                n541 = local write "Actual Field (T)"(w1107) -> ()
              }
            }
          }
        }
      }
      event "Go to Set": Value Change {
        n542 = event-data() -> ()  [unwired: 1 in, 6 out]
        n543 = local read "V/I (Ohm)"() -> (w1116:dbl)
        n544 = local read "B/V (T/V)"() -> (w1115:dbl)
        n545 = local read "Lock_in_Amplifier"() -> (w1112:refnum<visa-resource-name>)
        n546 = local read "Sweep Rate (T/min)"() -> (w1114:dbl)
        n547 = local read "Magnet"() -> (w1117:bool)
        n548 = call "Ramp_Field.vi"("Set Field (T) in"="Set Field (T)", "Sweep Rate (T/min)"=w1114, "V/I (Ohm)"=w1116, "error in (no error)"=w1118, "Magnet"=w1117, "B/V (T/V)"=w1115, "VISA Refnum in"=w1112) -> ("error out"=w1120:errorcluster, "Actual Voltage (V)"=w1110:dbl, "Set Field (T) out"=w1113:dbl)  [unwired: 2 in]
        n549 = local write "Actual B Field (T)"(w1113) -> ()
        n550 = local write "Actual Voltage (V)"(w1110) -> ()
      }
      event "Measure /Pause": Value Change {
        n551 = event-data() -> ("NewVal"=w1122:bool)  [unwired: 1 in, 5 out]
        n552 = local write "Measuring"(w1122) -> ()
      }
      event "Stop": Value Change {
        n553 = event-data() -> ()  [unwired: 1 in, 6 out]
        n554 = local read "Measuring"() -> (w1130:bool)
        n555 = case shown="True" w1130 {
          tunnel: w1129 -> [w1131 w1134]
          tunnel: [w1131 w1135] -> w1128
          frame False {
          }
          frame True {
            w1142 = FALSE ("Measuring")
            n556 = local read "SaveSweep"() -> (w1143:bool)
            n557 = local write "Measuring"(w1142) -> ()
            n558 = local write "Measure /Pause"(w1142) -> ()
            n559 = local read "Lock_in_Amplifier"() -> (w1136:refnum<visa-resource-name>)
            n560 = case shown="True" w1143 {
              frame False {
              }
              frame True {
                w1149 = 1 ("index (row)")
                w1150 = 0 ("index (row)")
                n561 = local read "Measurement File_average"() -> (w1162:path)
                n562 = local read "Averaged P(B)"() -> (w1151:dbl[][])
                n563 = local read "Averaged dt"() -> (w1153:dbl[][])
                n564 = local read "I(B) /Averaged/"() -> (w1161:cluster{"B array":dbl[], dbl[]}[])
                n565 = Index Array(array=w1153, index (row)=w1150) -> (element=w1152:dbl[])  [unwired: 1 in]
                n566 = Index Array(array=w1153, index (row)=w1149) -> (element=w1145:dbl[])  [unwired: 1 in]
                n567 = Index Array(array=w1161, index=1) -> (element=w1157:cluster{"B array":dbl[], dbl[]})
                n568 = Index Array(array=w1161, index=0) -> (element=w1158:cluster{"B array":dbl[], dbl[]})
                n569 = Unbundle(w1157) -> ("B array"=w1147:dbl[], w1146:dbl[])
                n570 = Unbundle(w1158) -> ("B array"=w1156:dbl[], w1155:dbl[])
                n571 = Index Array(array=w1151, index (row)=w1150) -> (element=w1148:dbl[])  [unwired: 1 in]
                n572 = Index Array(array=w1151, index (row)=w1149) -> (element=w1144:dbl[])  [unwired: 1 in]
                n573 = Build Array(w1156, w1155, w1152, w1148, w1147, w1146, w1145, w1144) -> (w1154:dbl[][])
                n574 = call-poly <vilib>:"Write Delimited Spreadsheet.vi"("file path (dialog if empty)"=w1162, "format (%.3f)"="%.5g", "2D data"=w1154, "append to file? (F)"=TRUE ("transpose? (F)"), "transpose? (F)"=TRUE ("append to file? (F)")) -> ()  [unwired: 9 in, 2 out]
              }
            }
            n575 = local read "V/I (Ohm)"() -> (w1140:dbl)
            n576 = local read "Sweep Rate (T/min)"() -> (w1139:dbl)
            n577 = local read "Set Field (T)"() -> (w1141:dbl)
            n578 = local read "B/V (T/V)"() -> (w1137:dbl)
            n579 = local read "Magnet"() -> (w1138:bool)
            n580 = call "Ramp_Field.vi"("Set Field (T) in"=w1141, "Sweep Rate (T/min)"=w1139, "V/I (Ohm)"=w1140, "error in (no error)"=w1134, "Magnet"=w1138, "B/V (T/V)"=w1137, "VISA Refnum in"=w1136) -> ("error out"=w1135:errorcluster, "Actual Voltage (V)"=w1132:dbl, "Set Field (T) out"=w1133:dbl)  [unwired: 2 in]
            n581 = local write "Actual B Field (T)"(w1133) -> ()
            n582 = local write "Actual Voltage (V)"(w1132) -> ()
          }
        }
      }
      event "Sweep": Value Change {
        n583 = event-data() -> ("NewVal"=w1169:bool)  [unwired: 1 in, 5 out]
        n584 = case shown="True" w1169 {
          frame False {
          }
          frame True {
            n585 = local read "Measurement File"() -> (w1170:path)
            n586 = Two Button Dialog(message="Do you want to create additional files for the sweeping measurements?" ("string"), 1:"No" ("F button name (\"Cancel\")"), 2:"Yes" ("T button name (\"OK\")")) -> (T button?=w1172:bool)
            n587 = case shown="True" w1172 {
              tunnel: w1170 -> [_ w1177]
              frame False {
                n588 = local write "SaveSweep"(FALSE ("SaveSweep")) -> ()
              }
              frame True {
                n589 = call "Create_sweep_files.vi"("Measurement File"=w1177) -> ("Path 3"=→"Measurement File_dn":path, "Path 2"=→"Measurement File_up":path, "Path"=→"Measurement File_average":path)  [unwired: 8 in]
                "SaveSweep" <- TRUE
              }
            }
          }
        }
      }
      event "Measure Noise": Value Change {
        n590 = event-data() -> ("NewVal"=w1184:bool)  [unwired: 1 in, 5 out]
        n591 = case shown="True" w1184 {
          frame False {
          }
          frame True {
            n592 = local read "Gain (V/A)"() -> (w1189:dbl)
            n593 = call "Noise_measurement.vi"("Gain (V/A)"=w1189, "Cycles"="Cycles", "Lower Cut-Off"="Cut-Off Frequency", "minimum value"="minimum value", "Filter On"="Filter On", "maximum value"="maximum value", "physical channels"="physical channels", "rate"="Rate", "samples per channel"="Samples per channel") -> ("Current (pA) Filtered"=→"Current (pA) Filtered":waveform(dbl), "PSD (pA/Hz^1/2) Peaks Removed"=→"PSD (pA/Hz^1/2) Peaks Removed":cluster{"f0":dbl, "df":dbl, "magnitude":dbl[]}, "Current (pA)"=→"Current (pA)":dbl[], "PSD (pA/Hz^1/2)"=→"PSD (pA/Hz^1/2)":cluster{"f0":dbl, "df":dbl, "magnitude":dbl[]})  [unwired: 3 in]
          }
        }
      }
      event "Calibrate": Value Change {
        n594 = event-data() -> ()  [unwired: 1 in, 6 out]
        n595 = case shown="True" "Calibrate" {
          frame False {
          }
          frame True {
            w1204 = dbl[] []
            n596 = while {
              shift-right: [w1237] -> w1202
              shift-left: dbl[][] [] -> [w1236]
              shift-right: [w1220] -> _
              shift-left: w1204 -> [w1232]
              shift-right: [w1229] -> _
              shift-left: w1204 -> [w1231]
              shift-right: [w1219] -> _
              shift-left: w1204 -> [w1230]
              shift-right: [w1211] -> _
              shift-left: 0.0 ("Set Field out") -> [w1210]
              stop <- w1233 stop-if-true
              n597 = call "Calibtarion.vi"("Dwell Time (ms)"="Dwell Time (ms)", "V array in (V)"=w1232, "I array in (A)"=w1230, "Collected array in"=w1236, "B array in (T)"=w1231, "Set Field (T)"=w1210, "dB"="dB") -> ("Best Linear Fit"=w1221:dbl[], "appended array"=→"appended array":dbl[][], "slope"=→"B/V (T/V)":dbl, "V array out (V)"=w1220:dbl[], "Boolean"=w1235:bool, "I array out (A)"=w1219:dbl[], "intercept 2"=→"I0 (A)":dbl, "Collected array out"=w1237:dbl[][], "intercept"=→"B0 (T)":dbl, "B array Out"=w1229:dbl[], "slope 2"=→"V/I (Ohm)":dbl, "Best Linear Fit 2"=w1226:dbl[], "Set Field out"=w1211:dbl)
              n598 = Bundle("I array out (A)"=w1219, "V array out (V)"=w1220) -> (w1228:T15)  [unwired: 1 in]
              n599 = Bundle("I array out (A)"=w1219, "Best Linear Fit"=w1221) -> (w1222:T16)  [unwired: 1 in]
              n600 = Bundle("V array out (V)"=w1220, "B array Out"=w1229) -> (w1224:T17)  [unwired: 1 in]
              n601 = Bundle("V array out (V)"=w1220, "Best Linear Fit 2"=w1226) -> (w1225:T18)  [unwired: 1 in]
              n602 = Or(x=w1235, y="stop 2") -> (x .or. y?=w1233:bool)
              n603 = Build Array(w1228, w1222) -> (→"V_I":T19)
              n604 = Build Array(w1224, w1225) -> (→"B_V":T20)
            }
            n605 = flat-sequence {
              tunnel: w1202 -> [w1208]
              frame #0 {
                n606 = Two Button Dialog(message="Do you want to save calibration file?") -> (T button?=w1207:bool)  [unwired: 2 in]
                n607 = case shown="True" w1207 {
                  tunnel: w1208 -> [_ w1209]
                  frame False {
                  }
                  frame True {
                    n608 = call-poly <vilib>:"Write Delimited Spreadsheet.vi"("2D data"=w1209) -> ()  [unwired: 13 in, 2 out]
                  }
                }
              }
            }
          }
        }
      }
      event "New Measurement File": Value Change {
        n609 = event-data() -> ()  [unwired: 1 in, 6 out]
        n610 = local read "Sweep"() -> (w1239:bool)
        n611 = Open/Create/Replace File(prompt="Please select measurement file\n", operation (0:open)=T5."replace or create with confirmation") -> (refnum out=w1245:refnum<file>)  [unwired: 4 in, 2 out]
        n612 = local write "refnum out"(w1245) -> ()
        n613 = Refnum to Path(1:w1245) -> (0:w1240:path)
        n614 = case shown="True" w1239 {
          tunnel: w1240 -> [_ w1248]
          frame False {
          }
          frame True {
            n615 = Two Button Dialog(message="Do you want to create additional files for the sweeping measurements?" ("string"), 1:"No" ("F button name (\"Cancel\")"), 2:"Yes" ("T button name (\"OK\")")) -> (T button?=w1250:bool)
            n616 = case shown="True" w1250 {
              tunnel: w1248 -> [_ w1258]
              frame False {
                n617 = local write "SaveSweep"(FALSE ("SaveSweep")) -> ()
              }
              frame True {
                n618 = call "Create_sweep_files.vi"("Measurement File"=w1258) -> ("Path 3"=w1255:path, "Path 2"=w1256:path, "Path"=w1257:path)  [unwired: 8 in]
                n619 = local write "Measurement File_dn"(w1255) -> ()
                n620 = local write "Measurement File_average"(w1257) -> ()
                n621 = local write "Measurement File_up"(w1256) -> ()
                n622 = local write "SaveSweep"(TRUE) -> ()
              }
            }
          }
        }
        n623 = local write "Measurement File"(w1240) -> ()
        n624 = local write "Offset?"(FALSE ("Offset?")) -> ()
        n625 = local write "First?"(TRUE ("First?")) -> ()
      }
      event "Heater On/Off": Value Change {
        n626 = event-data() -> ()  [unwired: 1 in, 6 out]
        n627 = case shown="False" "Heater On/Off" {
          tunnel: w1263 -> [w1268 w1274]
          tunnel: w1262 -> [w1266 w1275]
          tunnel: [w1265 w1273] -> w1261
          frame False {
            n628 = VISA Write(VISA resource name=w1268, write buffer="RANGE,1,0", error in (no error)=w1266) -> (error out=w1265:errorcluster)  [unwired: 2 out]
          }
          frame True {
            n629 = Number To Decimal String(number="Heater Range") -> (decimal integer string=w1271:string)  [unwired: 1 in]
            n630 = Concatenate Strings("RANGE,1," ("write buffer"), w1271) -> (w1269:string)
            n631 = VISA Write(VISA resource name=w1274, write buffer=w1269, error in (no error)=w1275) -> (error out=w1273:errorcluster)  [unwired: 2 out]
          }
        }
      }
      event "Set temperature (K)": Value Change {
        n632 = event-data() -> ()  [unwired: 1 in, 6 out]
        n633 = local read "Set temperature (K)"() -> (w1281:dbl)
        n634 = Number To Fractional String(number=w1281, precision (6)=i16 3) -> (F-format string=w1284:string)  [unwired: 2 in]
        n635 = Concatenate Strings("SETP 1," ("write buffer"), w1284) -> (w1282:string)
        n636 = VISA Write(VISA resource name=w1278, write buffer=w1282, error in (no error)=w1280) -> (error out=w1279:errorcluster)  [unwired: 2 out]
      }
      event "Temp Ramping Rate (K/min)": Value Change {
        n637 = event-data() -> ()  [unwired: 1 in, 6 out]
        n638 = local read "Temp Ramping Rate (K/min)"() -> (w1288:dbl)
        n639 = Number To Fractional String(number=w1288, precision (6)=i16 1) -> (F-format string=w1294:string)  [unwired: 2 in]
        n640 = Concatenate Strings("RAMP 1,1," ("string"), w1294) -> (w1293:string)
        n641 = VISA Write(VISA resource name=w1291, write buffer=w1293, error in (no error)=w1290) -> (error out=w1289:errorcluster)  [unwired: 2 out]
      }
      event "Heater Range": Value Change {
        n642 = event-data() -> ()  [unwired: 1 in, 6 out]
        n643 = local read "Heater On/Off"() -> (w1300:bool)
        n644 = case shown="True" w1300 {
          tunnel: w1299 -> [w1301 w1306]
          tunnel: [w1301 w1305] -> w1298
          tunnel: w1296 -> [_ w1304]
          frame False {
          }
          frame True {
            n645 = local read "Heater Range"() -> (w1302:enum16{"Off", "Low", "Medium", "High"})
            n646 = Number To Decimal String(number=w1302) -> (decimal integer string=w1308:string)  [unwired: 1 in]
            n647 = Concatenate Strings("RANGE,1," ("write buffer"), w1308) -> (w1307:string)
            n648 = VISA Write(VISA resource name=w1304, write buffer=w1307, error in (no error)=w1306) -> (error out=w1305:errorcluster)  [unwired: 2 out]
          }
        }
      }
    }
    n649 = Reciprocal(x="Sampling rate (Hz)") -> (1/x=w943:dbl)
    n650 = Multiply(x=w943, y=1000.0) -> (x*y=w941:dbl)
    n651 = Wait Until Next ms Multiple(millisecond multiple=w941) -> ()  [unwired: 1 out]
  }
  n652 = local read "Max Field (T)"() -> (w72:dbl)
  n653 = local read "Min Field (T)"() -> (w74:dbl)
  n654 = local read "dB (T)"() -> (w73:dbl)
  n655 = Divide(x=w72, y=w73) -> (x/y=w75:dbl)
  n656 = for {
    N: w75 -> [_]
    tunnel: w73 -> [w1313]
    tunnel: [w1310] -> w35 mode=indexing
    tunnel: w74 -> [w1311]
    tunnel: [0.0] -> _ mode=indexing
    i -> [w1314]
    n657 = Multiply(x=w1314, y=w1313) -> (x*y=w1312:dbl)
    n658 = Add(x=w1312, y=w1311) -> (x+y=w1310:dbl)
  }
  n659 = Multiply(x=w35, y=0.0) -> (x*y=w32:dbl[])
  n660 = Array Size(array=w32) -> (size(s)=w31:i32)
  n661 = Decrement(x=w31) -> (x-1=w30:i32)
  n662 = local write "B array"(w35) -> ()
  n663 = Array Subset(array=w32, length=w30) -> (w29:dbl[])  [unwired: 1 in]
  n664 = Build Array(w32, w32) -> (w33:dbl[][])
  n665 = local read "Max temperature (K)"() -> (w1:dbl)
  n666 = local read "Min Temperature (K)"() -> (w3:dbl)
  n667 = local write "Averaged I(B)"(w33) -> ()
  n668 = Build Array(w29, w29) -> (w28:dbl[][])
  n669 = Divide(x=w1, y="dt (K)") -> (x/y=w5:dbl)
  n670 = local write "Averaged P(B)"(w28) -> ()
  n671 = local write "Averaged dt"(w28) -> ()
  n672 = for {
    N: w5 -> [_]
    tunnel: "dt (K)" -> [w1319]
    tunnel: [w1316] -> w4 mode=indexing
    tunnel: w3 -> [w1317]
    tunnel: [0.0] -> _ mode=indexing
    i -> [w1320]
    n673 = Multiply(x=w1320, y=w1319) -> (x*y=w1318:dbl)
    n674 = Add(x=w1318, y=w1317) -> (x+y=w1316:dbl)
  }
  "T array" <- w4
  n675 = local read "Lake Shore"() -> (w85:refnum<visa-resource-name>)
  n676 = local read "IV converter"() -> (w101:refnum<visa-resource-name>)
  n677 = local read "Magnetic Field"() -> (w100:refnum<visa-resource-name>)
  n678 = VISA Close(VISA resource name=w101, error in (no error)=w103) -> (error out=w104:errorcluster)
  n679 = VISA Close(VISA resource name=w100, error in (no error)=w104) -> (error out=w102:errorcluster)
  n680 = Release Queue(queue=w108, error in (no error)=w102) -> (error out=w98:errorcluster)  [unwired: 1 in, 2 out]
  n681 = Merge Errors(w98, w97) -> (w99:errorcluster)
  n682 = VISA Close(VISA resource name=w85, error in (no error)=w99) -> (error out=w96:errorcluster)
  n683 = local read "refnum out"() -> (w94:refnum<file>)
  n684 = Close File(refnum=w94, error in=w96) -> (error out=w95:errorcluster)  [unwired: 1 out]
  n685 = call <vilib>:"Simple Error Handler.vi"("error in (no error)"=w95) -> ()  [unwired: 4 in, 5 out]
  "i" <- w65
  "j" <- w65
